vi "HandleObservation_001.vi"(8 "error in (no error)":errorcluster, 11 "S4ACS_GUI in":refnum<class "S4ACS_GUI.lvclass">) -> (0 "error out":errorcluster, 3 "S4ACS_GUI out":refnum<class "S4ACS_GUI.lvclass">)   [LabVIEW 2018, in "S4ACS_GUI.lvclass"]
uses:
  S4ACS_GUI.lvclass
  S4ACS_GUI.lvclass/S4ACS_GUI.ctl
  Instrument/Instrument.lvclass/Instrument.ctl
  Device/Optics/Optics.lvclass/Optics.ctl
  Device/Optics/Opt_Selector/Opt_Selector.lvclass
  C:/Users/observer/Desktop/Sparc4GUI/SPARC4_GUI/Device/Optics/Optics.lvclass
  Instrument/Instrument.lvclass
  StateMachine/State Machine.lvclass
  SyncBox/Sync Box.lvclass
  Trigger/Trigger.lvclass
  Acquisition/Acquisition.lvclass
  Channel/Channel.lvclass
  Device/Optics/Optics.lvclass
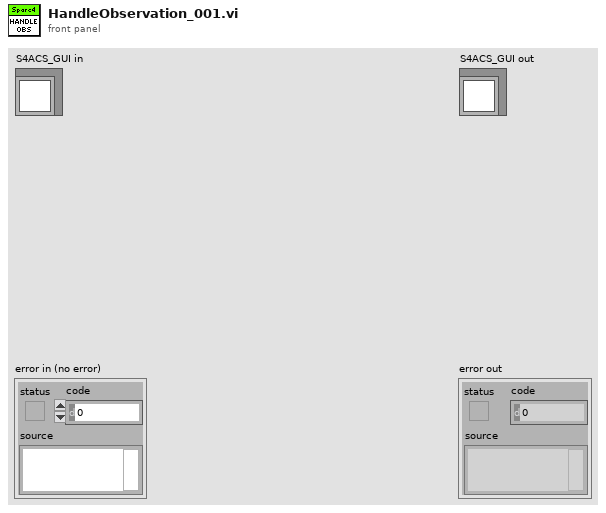
[diagram p1: front panel]
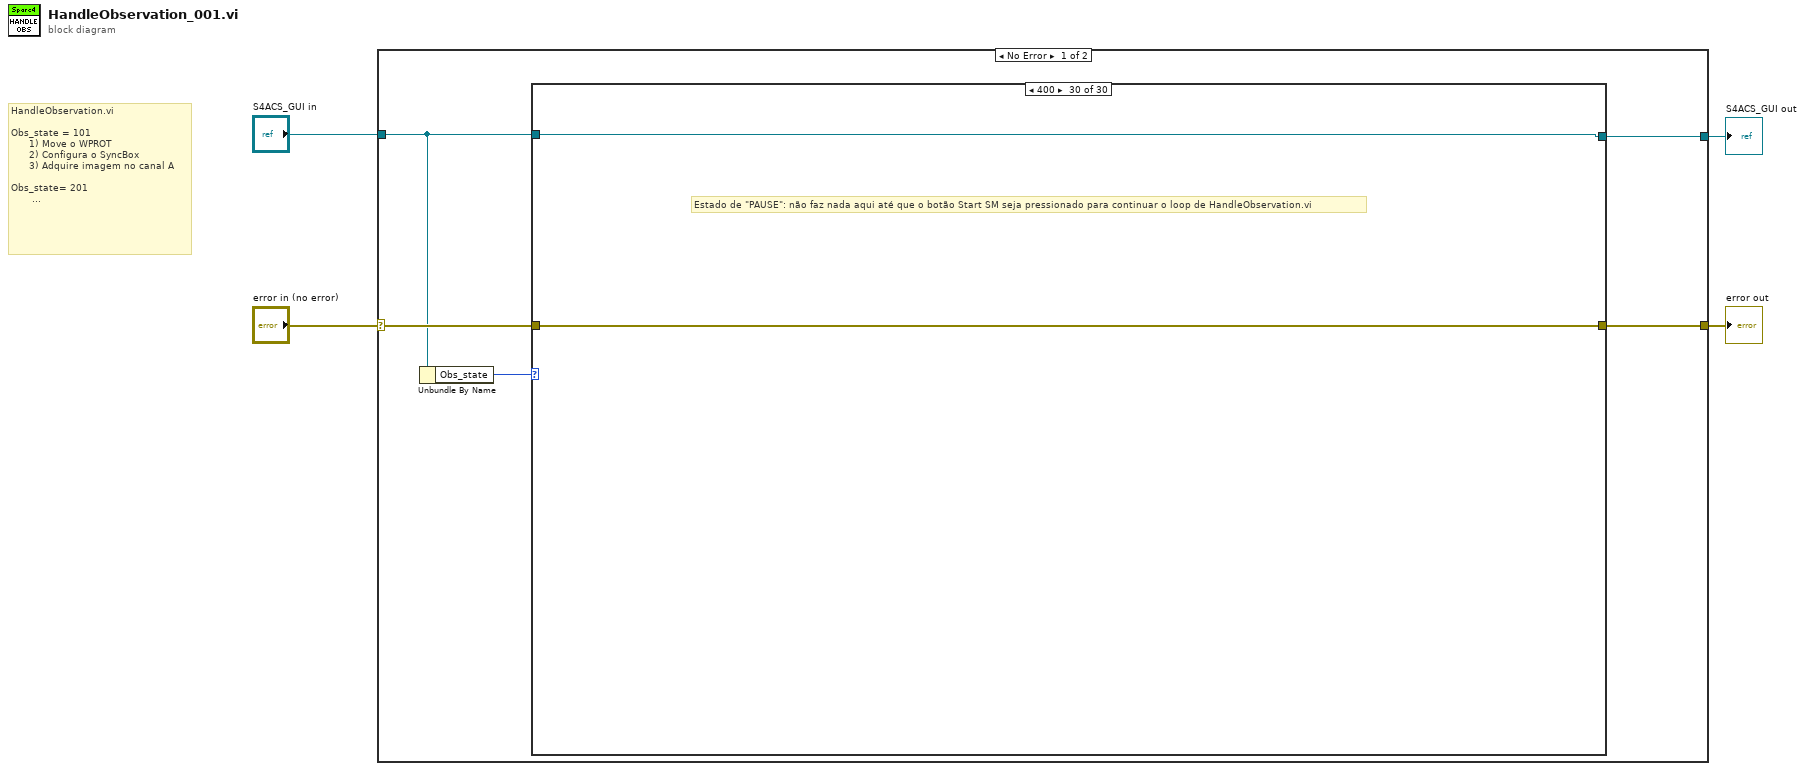
[diagram p0: block diagram]
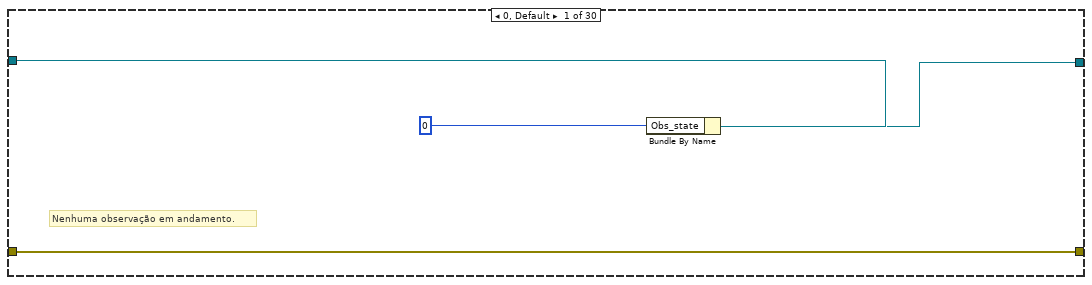
[diagram p2: hidden frame]
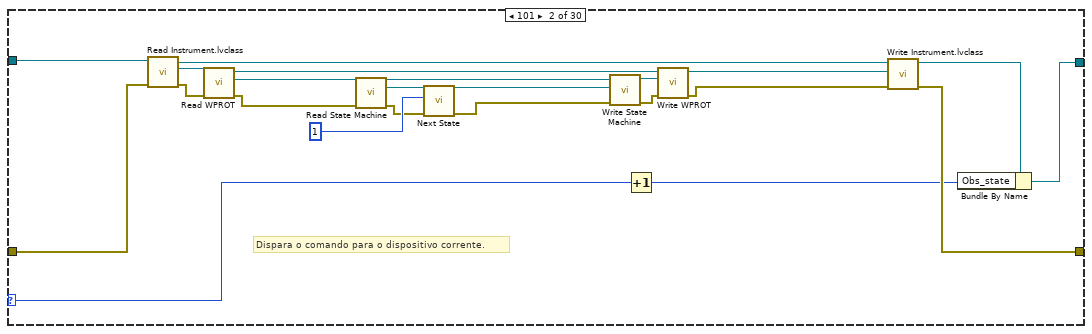
[diagram p3: hidden frame]
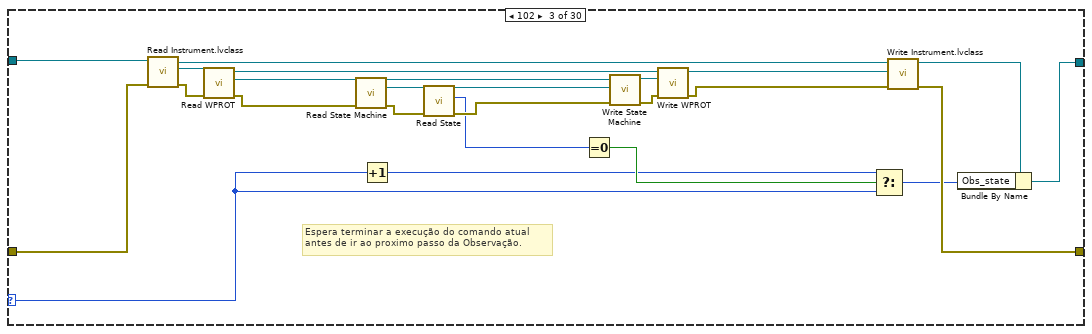
[diagram p4: hidden frame]
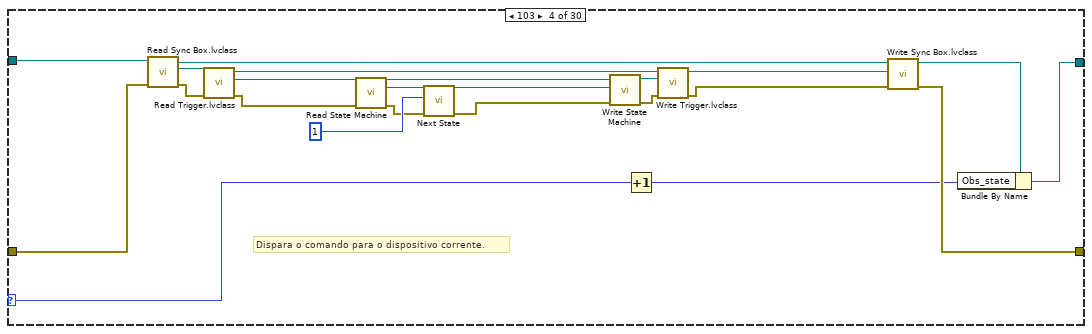
[diagram p5: hidden frame]
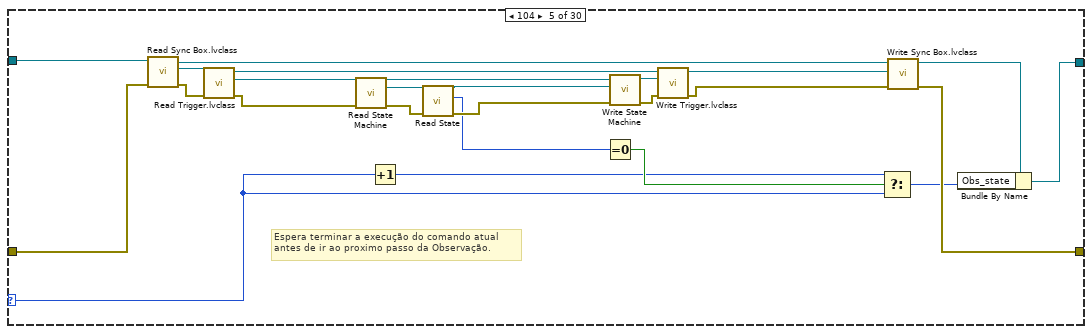
[diagram p6: hidden frame]
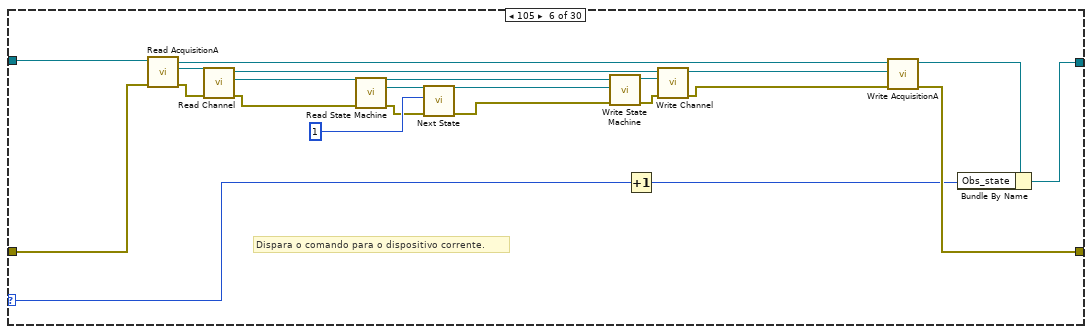
[diagram p7: hidden frame]
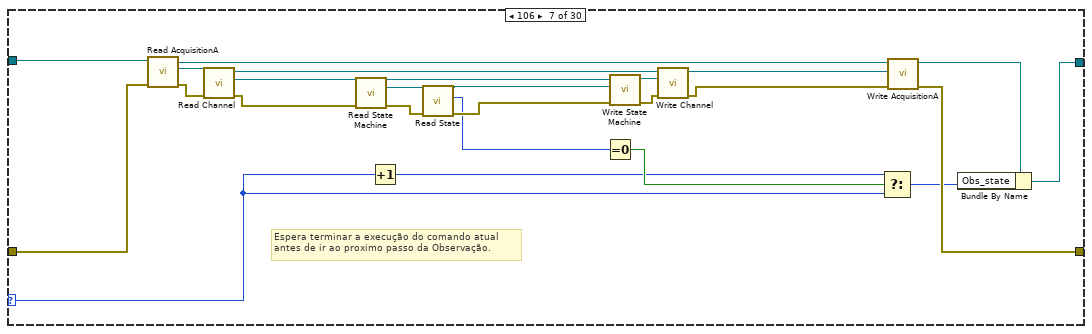
[diagram p8: hidden frame]
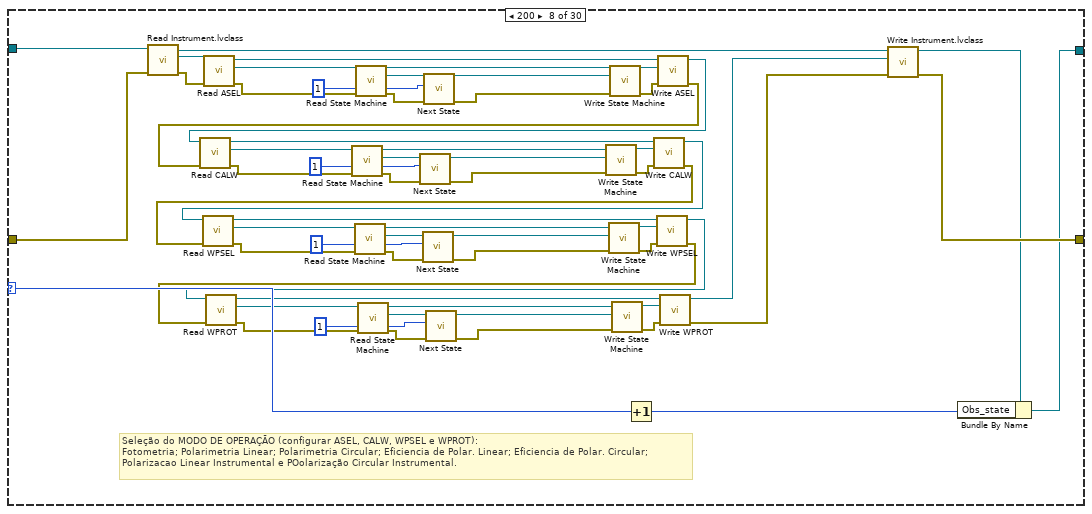
[diagram p9: hidden frame]
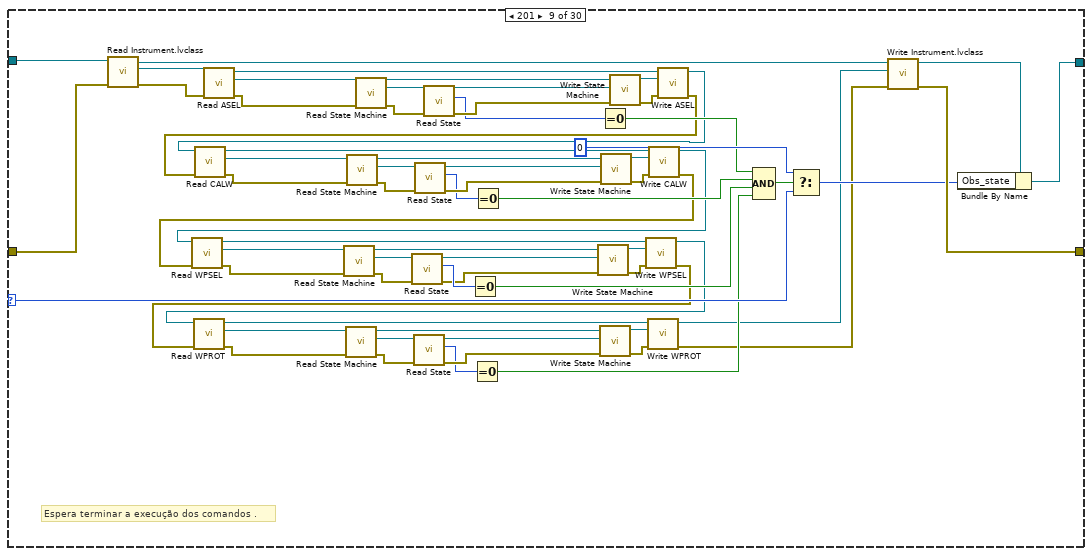
[diagram p10: hidden frame]
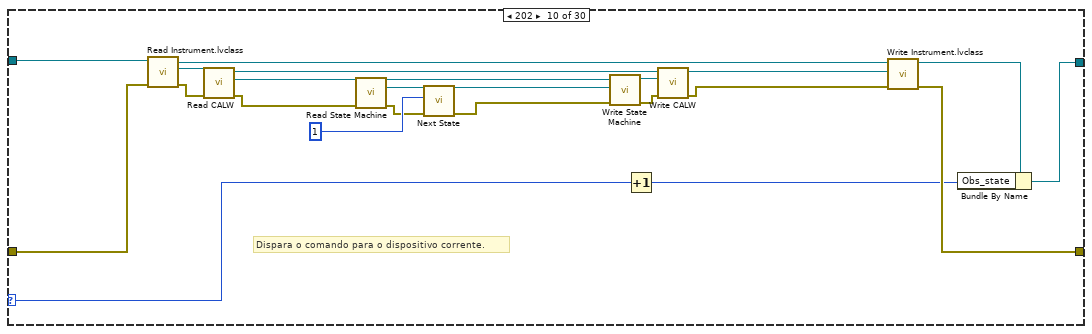
[diagram p11: hidden frame]
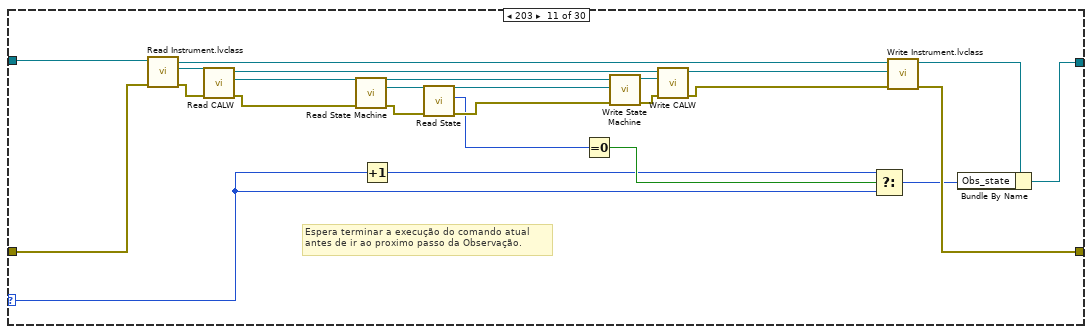
[diagram p12: hidden frame]
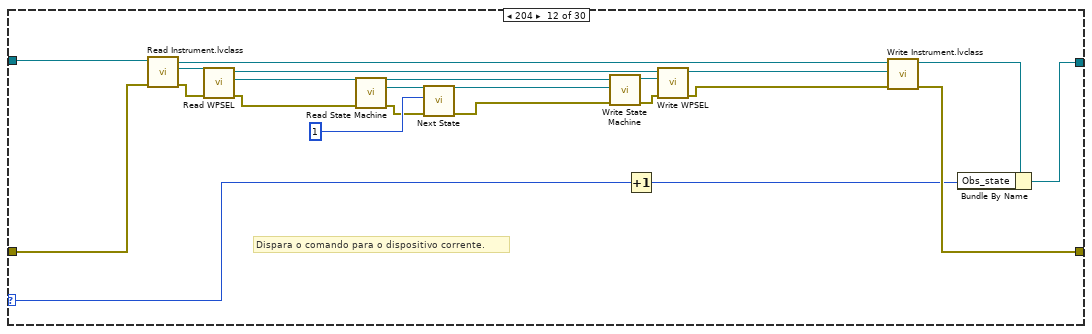
[diagram p13: hidden frame]
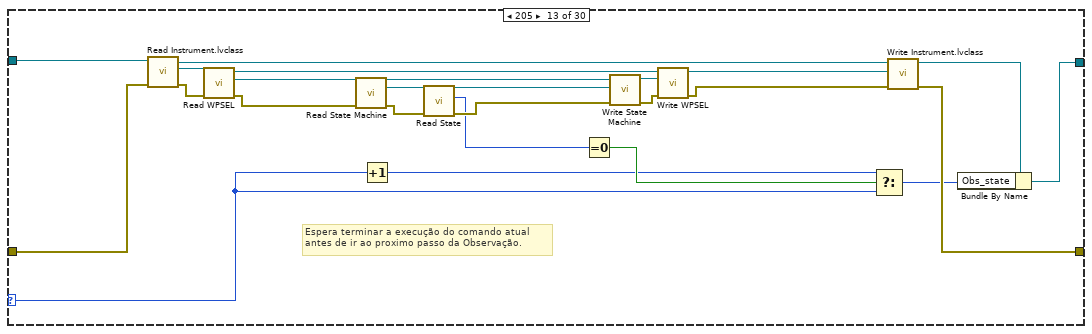
[diagram p14: hidden frame]
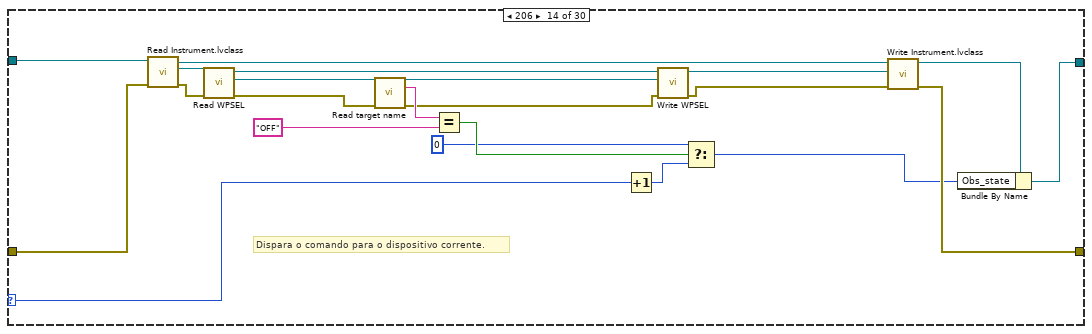
[diagram p15: hidden frame]
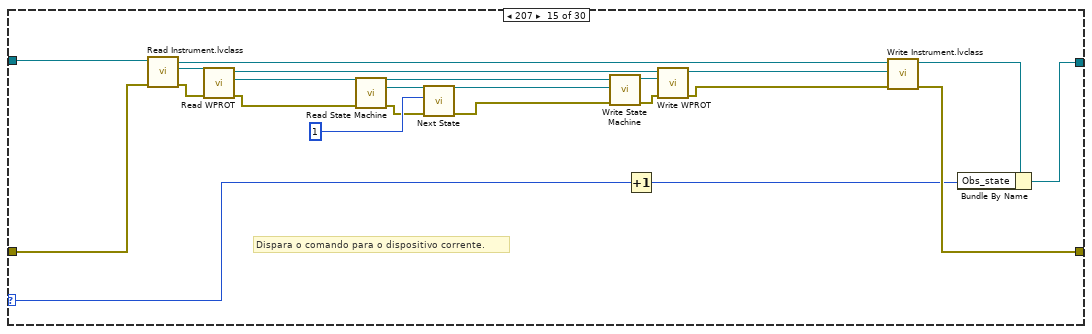
[diagram p16: hidden frame]
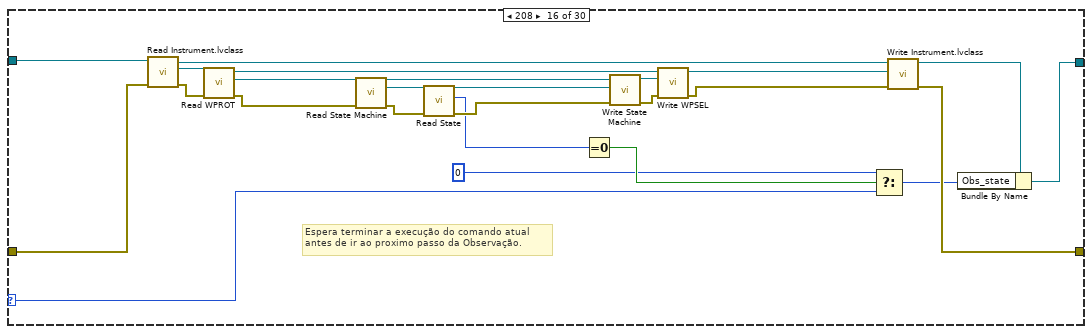
[diagram p17: hidden frame]
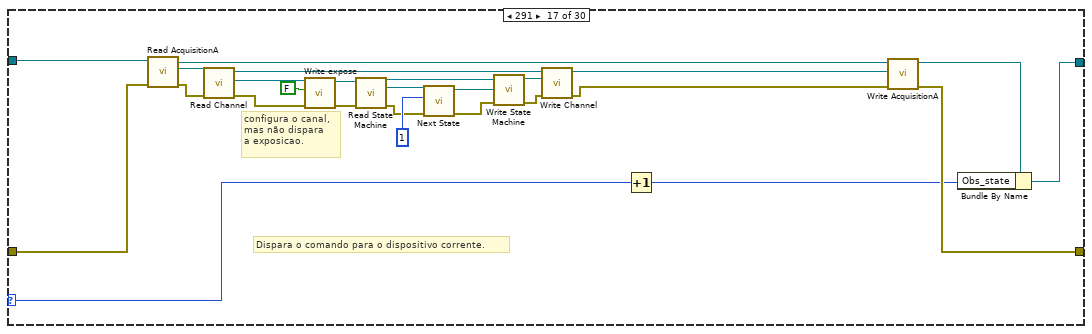
[diagram p18: hidden frame]
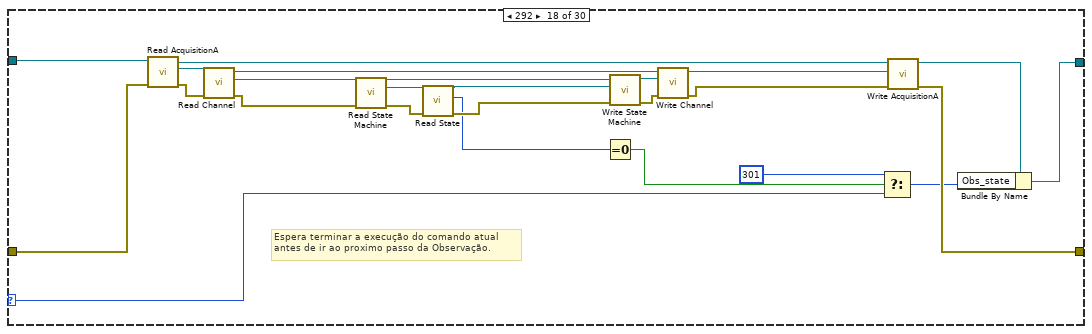
[diagram p19: hidden frame]
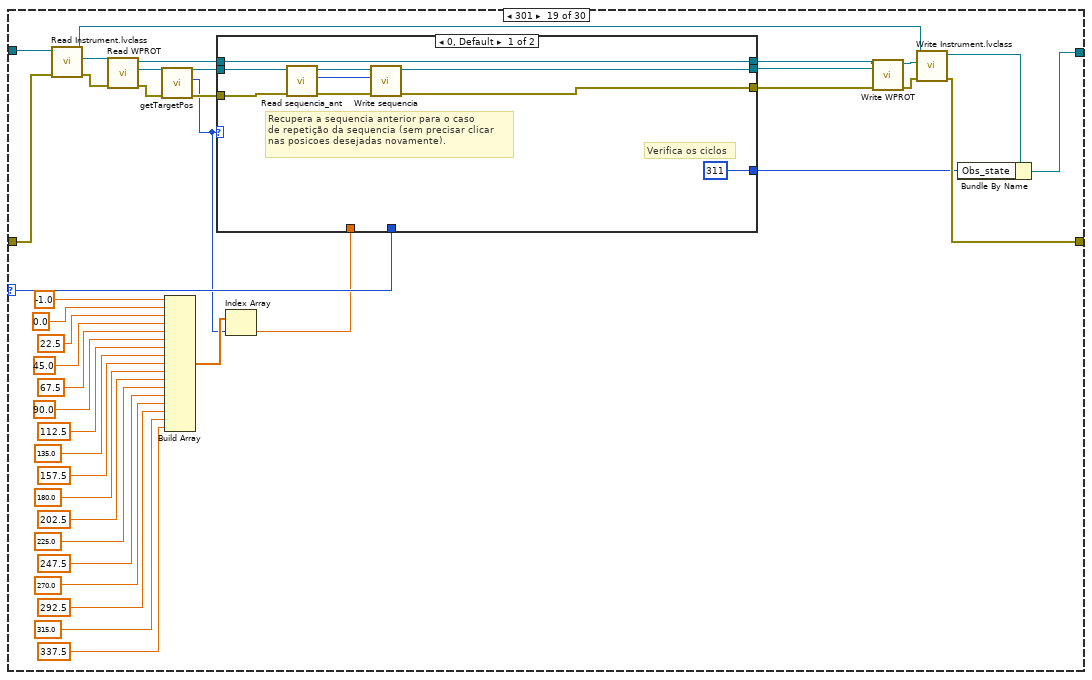
[diagram p20: hidden frame]
diagram:
  # "HandleObservation.vi\n\nObs_state = 101\n      1) Move o WPROT\n      2) Configura o SyncBox\n      3) Adquire imagem no canal A\n\nObs_state= 201\n       ..."
  n1 = case shown="No Error" "error in (no error)" {
    selector: "error in (no error)" -> [w8 w824]
    tunnel: [w7 w824] -> w3
    tunnel: [w9 w823] -> w1
    tunnel: "S4ACS_GUI in" -> [w6 w823]
    frame No Error {
      n2 = Unbundle By Name(w6) -> ("Obs_state"=w5:u32)
      n3 = case shown="400" w5 {
        selector: w5 -> [_ w16 w38 w64 w86 w112 w134 w202 w265 w290 w312 w338 w360 w395 w408 w430 w463 w482 w536 w582 w604 w636 w655 w686 w705 w734 w753 w778 _ _]
        tunnel: w6 -> [w12 w30 w55 w78 w103 w126 w151 w216 w283 w304 w329 w352 w377 w399 w422 w447 w473 w498 w540 w597 w621 w648 w672 w698 w722 w746 w770 w795 w815 w822]
        tunnel: [w10 w14 w42 w62 w94 w110 w142 w200 w270 w288 w316 w336 w364 w394 w406 w434 w461 w489 w534 w586 w612 w634 w663 w684 w713 w732 w761 w786 w811 w822] -> w9
        tunnel: w8 -> [w13 w29 w54 w77 w102 w125 w150 w215 w282 w303 w328 w351 w376 w398 w421 w446 w472 w497 w539 w596 w620 w647 w671 w697 w721 w745 w769 w794 w814 w821]
        tunnel: [w13 w28 w53 w76 w101 w124 w149 w214 w281 w302 w327 w350 w375 w397 w420 w445 w471 w496 w538 w595 w619 w646 w670 w696 w720 w744 w768 w793 w813 w821] -> w7
        frame 0, Default {
          # "Nenhuma observação em andamento."
          n4 = Bundle By Name(cluster=w12, "Obs_state"=u32 0) -> (w10:refnum<class "S4ACS_GUI.lvclass">)
        }
        frame 101 {
          # "Dispara o comando para o dispositivo corrente."
          n5 = call "Read Instrument.lvclass.vi"("error in (no error)"=w29, "S4ACS_GUI in"=w30) -> ("error out"=w35:errorcluster, "Instrument.lvclass"=w36:refnum<class "Instrument.lvclass">, "S4ACS_GUI out"=w32:refnum<class "S4ACS_GUI.lvclass">)  [unwired: 7 in]
          n6 = call "Read WPROT.vi"("error in (no error)"=w35, "Instrument in"=w36) -> ("error out"=w22:errorcluster, "Opt_Selector.lvclass"=w21:refnum<class "Opt_Selector.lvclass">, "Instrument out"=w34:refnum<class "Instrument.lvclass">)  [unwired: 7 in]
          n7 = call-dynamic "Read State Machine.vi"("error in (no error)"=w22, "Device in"=w21) -> ("error out"=w25:errorcluster, "State Machine.lvclass"=w27:refnum<class "State Machine.lvclass">, "Device out"=w19:refnum<class "Opt_Selector.lvclass">)  [unwired: 7 in]
          n8 = call "Next State.vi"("error in (no error)"=w25, "New_State"=1, "State Machine in"=w27) -> ("error out"=w24:errorcluster, "State Machine out"=w23:refnum<class "State Machine.lvclass">)  [unwired: 7 in]
          n9 = call-dynamic "Write State Machine.vi"("error in (no error)"=w24, "State Machine.lvclass"=w23, "Device in"=w19) -> ("error out"=w18:errorcluster, "Device out"=w20:refnum<class "Opt_Selector.lvclass">)  [unwired: 7 in]
          n10 = Increment(x=w16) -> (x+1=w15:u32)
          n11 = call "Write WPROT.vi"("error in (no error)"=w18, "Opt_Selector.lvclass"=w20, "Instrument in"=w34) -> ("error out"=w31:errorcluster, "Instrument out"=w33:refnum<class "Instrument.lvclass">)  [unwired: 7 in]
          n12 = call "Write Instrument.lvclass.vi"("error in (no error)"=w31, "Instrument.lvclass"=w33, "S4ACS_GUI in"=w32) -> ("error out"=w28:errorcluster, "S4ACS_GUI out"=w17:refnum<class "S4ACS_GUI.lvclass">)  [unwired: 7 in]
          n13 = Bundle By Name(cluster=w17, "Obs_state"=w15) -> (w14:refnum<class "S4ACS_GUI.lvclass">)
        }
        frame 102 {
          # "Espera terminar a execução do comando atual \nantes de ir ao proximo passo da Observação."
          n14 = call "Read Instrument.lvclass.vi"("error in (no error)"=w54, "S4ACS_GUI in"=w55) -> ("error out"=w60:errorcluster, "Instrument.lvclass"=w61:refnum<class "Instrument.lvclass">, "S4ACS_GUI out"=w57:refnum<class "S4ACS_GUI.lvclass">)  [unwired: 7 in]
          n15 = call "Read WPROT.vi"("error in (no error)"=w60, "Instrument in"=w61) -> ("error out"=w48:errorcluster, "Opt_Selector.lvclass"=w47:refnum<class "Opt_Selector.lvclass">, "Instrument out"=w59:refnum<class "Instrument.lvclass">)  [unwired: 7 in]
          n16 = call-dynamic "Read State Machine.vi"("error in (no error)"=w48, "Device in"=w47) -> ("error out"=w51:errorcluster, "State Machine.lvclass"=w52:refnum<class "State Machine.lvclass">, "Device out"=w45:refnum<class "Opt_Selector.lvclass">)  [unwired: 7 in]
          n17 = Increment(x=w38) -> (x+1=w37:u32)
          n18 = call-dynamic "Read State.vi"("error in (no error)"=w51, "State Machine in"=w52) -> ("error out"=w50:errorcluster, "State"=w40:i32, "State Machine out"=w49:refnum<class "State Machine.lvclass">)  [unwired: 7 in]
          n19 = Equal To 0?(x=w40) -> (x = 0?=w41:bool)
          n20 = call-dynamic "Write State Machine.vi"("error in (no error)"=w50, "State Machine.lvclass"=w49, "Device in"=w45) -> ("error out"=w44:errorcluster, "Device out"=w46:refnum<class "Opt_Selector.lvclass">)  [unwired: 7 in]
          n21 = call "Write WPROT.vi"("error in (no error)"=w44, "Opt_Selector.lvclass"=w46, "Instrument in"=w59) -> ("error out"=w56:errorcluster, "Instrument out"=w58:refnum<class "Instrument.lvclass">)  [unwired: 7 in]
          n22 = Select(t=w37, s=w41, f=w38) -> (s? t:f=w39:u32)
          n23 = call "Write Instrument.lvclass.vi"("error in (no error)"=w56, "Instrument.lvclass"=w58, "S4ACS_GUI in"=w57) -> ("error out"=w53:errorcluster, "S4ACS_GUI out"=w43:refnum<class "S4ACS_GUI.lvclass">)  [unwired: 7 in]
          n24 = Bundle By Name(cluster=w43, "Obs_state"=w39) -> (w42:refnum<class "S4ACS_GUI.lvclass">)
        }
        frame 103 {
          # "Dispara o comando para o dispositivo corrente."
          n25 = call-dynamic "Read Sync Box.lvclass.vi"("error in (no error)"=w77, "SPARC4_AC in"=w78) -> ("error out"=w83:errorcluster, "Sync Box.lvclass"=w84:refnum<class "Sync Box.lvclass">, "SPARC4_AC out"=w80:refnum<class "S4ACS_GUI.lvclass">)  [unwired: 7 in]
          n26 = call-dynamic "Read Trigger.lvclass.vi"("error in (no error)"=w83, "Sync Box in"=w84) -> ("error out"=w70:errorcluster, "Trigger.lvclass"=w69:refnum<class "Trigger.lvclass">, "Sync Box out"=w82:refnum<class "Sync Box.lvclass">)  [unwired: 7 in]
          n27 = call-dynamic "Read State Machine.vi"("error in (no error)"=w70, "Device in"=w69) -> ("error out"=w73:errorcluster, "State Machine.lvclass"=w75:refnum<class "State Machine.lvclass">, "Device out"=w67:refnum<class "Trigger.lvclass">)  [unwired: 7 in]
          n28 = call "Next State.vi"("error in (no error)"=w73, "New_State"=1, "State Machine in"=w75) -> ("error out"=w72:errorcluster, "State Machine out"=w71:refnum<class "State Machine.lvclass">)  [unwired: 7 in]
          n29 = call-dynamic "Write State Machine.vi"("error in (no error)"=w72, "State Machine.lvclass"=w71, "Device in"=w67) -> ("error out"=w66:errorcluster, "Device out"=w68:refnum<class "Trigger.lvclass">)  [unwired: 7 in]
          n30 = Increment(x=w64) -> (x+1=w63:u32)
          n31 = call-dynamic "Write Trigger.lvclass.vi"("error in (no error)"=w66, "Trigger.lvclass"=w68, "Sync Box in"=w82) -> ("error out"=w79:errorcluster, "Sync Box out"=w81:refnum<class "Sync Box.lvclass">)  [unwired: 7 in]
          n32 = call-dynamic "Write Sync Box.lvclass.vi"("error in (no error)"=w79, "Sync Box.lvclass"=w81, "SPARC4_AC in"=w80) -> ("error out"=w76:errorcluster, "SPARC4_AC out"=w65:refnum<class "S4ACS_GUI.lvclass">)  [unwired: 7 in]
          n33 = Bundle By Name(cluster=w65, "Obs_state"=w63) -> (w62:refnum<class "S4ACS_GUI.lvclass">)
        }
        frame 104 {
          # "Espera terminar a execução do comando atual \nantes de ir ao proximo passo da Observação."
          n34 = call-dynamic "Read Sync Box.lvclass.vi"("error in (no error)"=w102, "SPARC4_AC in"=w103) -> ("error out"=w108:errorcluster, "Sync Box.lvclass"=w109:refnum<class "Sync Box.lvclass">, "SPARC4_AC out"=w105:refnum<class "S4ACS_GUI.lvclass">)  [unwired: 7 in]
          n35 = call-dynamic "Read Trigger.lvclass.vi"("error in (no error)"=w108, "Sync Box in"=w109) -> ("error out"=w100:errorcluster, "Trigger.lvclass"=w99:refnum<class "Trigger.lvclass">, "Sync Box out"=w107:refnum<class "Sync Box.lvclass">)  [unwired: 7 in]
          n36 = call-dynamic "Read State Machine.vi"("error in (no error)"=w100, "Device in"=w99) -> ("error out"=w91:errorcluster, "State Machine.lvclass"=w93:refnum<class "State Machine.lvclass">, "Device out"=w97:refnum<class "Trigger.lvclass">)  [unwired: 7 in]
          n37 = Increment(x=w86) -> (x+1=w88:u32)
          n38 = call-dynamic "Read State.vi"("error in (no error)"=w91, "State Machine in"=w93) -> ("error out"=w90:errorcluster, "State"=w85:i32, "State Machine out"=w92:refnum<class "State Machine.lvclass">)  [unwired: 7 in]
          n39 = Equal To 0?(x=w85) -> (x = 0?=w89:bool)
          n40 = call-dynamic "Write State Machine.vi"("error in (no error)"=w90, "State Machine.lvclass"=w92, "Device in"=w97) -> ("error out"=w96:errorcluster, "Device out"=w98:refnum<class "Trigger.lvclass">)  [unwired: 7 in]
          n41 = call-dynamic "Write Trigger.lvclass.vi"("error in (no error)"=w96, "Trigger.lvclass"=w98, "Sync Box in"=w107) -> ("error out"=w104:errorcluster, "Sync Box out"=w106:refnum<class "Sync Box.lvclass">)  [unwired: 7 in]
          n42 = Select(t=w88, s=w89, f=w86) -> (s? t:f=w87:u32)
          n43 = call-dynamic "Write Sync Box.lvclass.vi"("error in (no error)"=w104, "Sync Box.lvclass"=w106, "SPARC4_AC in"=w105) -> ("error out"=w101:errorcluster, "SPARC4_AC out"=w95:refnum<class "S4ACS_GUI.lvclass">)  [unwired: 7 in]
          n44 = Bundle By Name(cluster=w95, "Obs_state"=w87) -> (w94:refnum<class "S4ACS_GUI.lvclass">)
        }
        frame 105 {
          # "Dispara o comando para o dispositivo corrente."
          n45 = call-dynamic "Read AcquisitionA.vi"("error in (no error)"=w125, "S4ACS_GUI in"=w126) -> ("error out"=w131:errorcluster, "Acquisition.lvclass"=w132:refnum<class "Acquisition.lvclass">, "S4ACS_GUI out"=w128:refnum<class "S4ACS_GUI.lvclass">)  [unwired: 7 in]
          n46 = call-dynamic "Read Channel.vi"("error in (no error)"=w131, "Acquisition in"=w132) -> ("error out"=w118:errorcluster, "Channel.lvclass"=w117:refnum<class "Channel.lvclass">, "Acquisition out"=w130:refnum<class "Acquisition.lvclass">)  [unwired: 7 in]
          n47 = call-dynamic "Read State Machine.vi"("error in (no error)"=w118, "Device in"=w117) -> ("error out"=w121:errorcluster, "State Machine.lvclass"=w123:refnum<class "State Machine.lvclass">, "Device out"=w115:refnum<class "Channel.lvclass">)  [unwired: 7 in]
          n48 = call "Next State.vi"("error in (no error)"=w121, "New_State"=1, "State Machine in"=w123) -> ("error out"=w120:errorcluster, "State Machine out"=w119:refnum<class "State Machine.lvclass">)  [unwired: 7 in]
          n49 = call-dynamic "Write State Machine.vi"("error in (no error)"=w120, "State Machine.lvclass"=w119, "Device in"=w115) -> ("error out"=w114:errorcluster, "Device out"=w116:refnum<class "Channel.lvclass">)  [unwired: 7 in]
          n50 = Increment(x=w112) -> (x+1=w111:u32)
          n51 = call-dynamic "Write Channel.vi"("error in (no error)"=w114, "Channel.lvclass"=w116, "Acquisition in"=w130) -> ("error out"=w127:errorcluster, "Acquisition out"=w129:refnum<class "Acquisition.lvclass">)  [unwired: 7 in]
          n52 = call-dynamic "Write AcquisitionA.vi"("error in (no error)"=w127, "Acquisition.lvclass"=w129, "S4ACS_GUI in"=w128) -> ("error out"=w124:errorcluster, "S4ACS_GUI out"=w113:refnum<class "S4ACS_GUI.lvclass">)  [unwired: 7 in]
          n53 = Bundle By Name(cluster=w113, "Obs_state"=w111) -> (w110:refnum<class "S4ACS_GUI.lvclass">)
        }
        frame 106 {
          # "Espera terminar a execução do comando atual \nantes de ir ao proximo passo da Observação."
          n54 = call-dynamic "Read AcquisitionA.vi"("error in (no error)"=w150, "S4ACS_GUI in"=w151) -> ("error out"=w156:errorcluster, "Acquisition.lvclass"=w157:refnum<class "Acquisition.lvclass">, "S4ACS_GUI out"=w153:refnum<class "S4ACS_GUI.lvclass">)  [unwired: 7 in]
          n55 = call-dynamic "Read Channel.vi"("error in (no error)"=w156, "Acquisition in"=w157) -> ("error out"=w148:errorcluster, "Channel.lvclass"=w147:refnum<class "Channel.lvclass">, "Acquisition out"=w155:refnum<class "Acquisition.lvclass">)  [unwired: 7 in]
          n56 = call-dynamic "Read State Machine.vi"("error in (no error)"=w148, "Device in"=w147) -> ("error out"=w139:errorcluster, "State Machine.lvclass"=w141:refnum<class "State Machine.lvclass">, "Device out"=w145:refnum<class "Channel.lvclass">)  [unwired: 7 in]
          n57 = Increment(x=w134) -> (x+1=w136:u32)
          n58 = call-dynamic "Read State.vi"("error in (no error)"=w139, "State Machine in"=w141) -> ("error out"=w138:errorcluster, "State"=w133:i32, "State Machine out"=w140:refnum<class "State Machine.lvclass">)  [unwired: 7 in]
          n59 = Equal To 0?(x=w133) -> (x = 0?=w137:bool)
          n60 = call-dynamic "Write State Machine.vi"("error in (no error)"=w138, "State Machine.lvclass"=w140, "Device in"=w145) -> ("error out"=w144:errorcluster, "Device out"=w146:refnum<class "Channel.lvclass">)  [unwired: 7 in]
          n61 = call-dynamic "Write Channel.vi"("error in (no error)"=w144, "Channel.lvclass"=w146, "Acquisition in"=w155) -> ("error out"=w152:errorcluster, "Acquisition out"=w154:refnum<class "Acquisition.lvclass">)  [unwired: 7 in]
          n62 = Select(t=w136, s=w137, f=w134) -> (s? t:f=w135:u32)
          n63 = call-dynamic "Write AcquisitionA.vi"("error in (no error)"=w152, "Acquisition.lvclass"=w154, "S4ACS_GUI in"=w153) -> ("error out"=w149:errorcluster, "S4ACS_GUI out"=w143:refnum<class "S4ACS_GUI.lvclass">)  [unwired: 7 in]
          n64 = Bundle By Name(cluster=w143, "Obs_state"=w135) -> (w142:refnum<class "S4ACS_GUI.lvclass">)
        }
        frame 200 {
          # "Seleção do MODO DE OPERAÇÃO (configurar ASEL, CALW, WPSEL e WPROT): \nFotometria; Polarimetria Linear; Polarimetria Circular; Eficiencia de Polar. Linear; Eficiencia de Polar. Circular;\nPolarizacao Linear Instrumental e POolarização Circular Instrumental."
          n65 = call "Read Instrument.lvclass.vi"("error in (no error)"=w215, "S4ACS_GUI in"=w216) -> ("error out"=w219:errorcluster, "Instrument.lvclass"=w179:refnum<class "Instrument.lvclass">, "S4ACS_GUI out"=w217:refnum<class "S4ACS_GUI.lvclass">)  [unwired: 7 in]
          n66 = call "Read ASEL.vi"("error in (no error)"=w219, "Instrument in"=w179) -> ("error out"=w208:errorcluster, "Opt_Selector.lvclass"=w207:refnum<class "Opt_Selector.lvclass">, "Instrument out"=w218:refnum<class "Instrument.lvclass">)  [unwired: 7 in]
          n67 = call-dynamic "Read State Machine.vi"("error in (no error)"=w208, "Device in"=w207) -> ("error out"=w211:errorcluster, "State Machine.lvclass"=w213:refnum<class "State Machine.lvclass">, "Device out"=w205:refnum<class "Opt_Selector.lvclass">)  [unwired: 7 in]
          n68 = call "Next State.vi"("error in (no error)"=w211, "New_State"=1, "State Machine in"=w213) -> ("error out"=w210:errorcluster, "State Machine out"=w209:refnum<class "State Machine.lvclass">)  [unwired: 7 in]
          n69 = call-dynamic "Write State Machine.vi"("error in (no error)"=w210, "State Machine.lvclass"=w209, "Device in"=w205) -> ("error out"=w204:errorcluster, "Device out"=w206:refnum<class "Opt_Selector.lvclass">)  [unwired: 7 in]
          n70 = Increment(x=w202) -> (x+1=w201:u32)
          n71 = call "Write ASEL.vi"("error in (no error)"=w204, "Opt_Selector.lvclass"=w206, "Instrument in"=w218) -> ("error out"=w160:errorcluster, "Instrument out"=w178:refnum<class "Instrument.lvclass">)  [unwired: 7 in]
          n72 = call "Read CALW.vi"("error in (no error)"=w160, "Instrument in"=w178) -> ("error out"=w195:errorcluster, "Opt_Selector.lvclass"=w196:refnum<class "Opt_Selector.lvclass">, "Instrument out"=w177:refnum<class "Instrument.lvclass">)  [unwired: 7 in]
          n73 = call-dynamic "Read State Machine.vi"("error in (no error)"=w195, "Device in"=w196) -> ("error out"=w192:errorcluster, "State Machine.lvclass"=w190:refnum<class "State Machine.lvclass">, "Device out"=w198:refnum<class "Opt_Selector.lvclass">)  [unwired: 7 in]
          n74 = call "Next State.vi"("error in (no error)"=w192, "New_State"=1, "State Machine in"=w190) -> ("error out"=w193:errorcluster, "State Machine out"=w194:refnum<class "State Machine.lvclass">)  [unwired: 7 in]
          n75 = call-dynamic "Write State Machine.vi"("error in (no error)"=w193, "State Machine.lvclass"=w194, "Device in"=w198) -> ("error out"=w199:errorcluster, "Device out"=w197:refnum<class "Opt_Selector.lvclass">)  [unwired: 7 in]
          n76 = call "Write CALW.vi"("error in (no error)"=w199, "Opt_Selector.lvclass"=w197, "Instrument in"=w177) -> ("error out"=w159:errorcluster, "Instrument out"=w176:refnum<class "Instrument.lvclass">)  [unwired: 7 in]
          n77 = call "Read WPSEL.vi"("error in (no error)"=w159, "Instrument in"=w176) -> ("error out"=w184:errorcluster, "Opt_Selector.lvclass"=w183:refnum<class "Opt_Selector.lvclass">, "Instrument out"=w175:refnum<class "Instrument.lvclass">)  [unwired: 7 in]
          n78 = call-dynamic "Read State Machine.vi"("error in (no error)"=w184, "Device in"=w183) -> ("error out"=w187:errorcluster, "State Machine.lvclass"=w189:refnum<class "State Machine.lvclass">, "Device out"=w181:refnum<class "Opt_Selector.lvclass">)  [unwired: 7 in]
          n79 = call "Next State.vi"("error in (no error)"=w187, "New_State"=1, "State Machine in"=w189) -> ("error out"=w186:errorcluster, "State Machine out"=w185:refnum<class "State Machine.lvclass">)  [unwired: 7 in]
          n80 = call-dynamic "Write State Machine.vi"("error in (no error)"=w186, "State Machine.lvclass"=w185, "Device in"=w181) -> ("error out"=w180:errorcluster, "Device out"=w182:refnum<class "Opt_Selector.lvclass">)  [unwired: 7 in]
          n81 = call "Write WPSEL.vi"("error in (no error)"=w180, "Opt_Selector.lvclass"=w182, "Instrument in"=w175) -> ("error out"=w158:errorcluster, "Instrument out"=w164:refnum<class "Instrument.lvclass">)  [unwired: 7 in]
          n82 = call "Read WPROT.vi"("error in (no error)"=w158, "Instrument in"=w164) -> ("error out"=w170:errorcluster, "Opt_Selector.lvclass"=w171:refnum<class "Opt_Selector.lvclass">, "Instrument out"=w163:refnum<class "Instrument.lvclass">)  [unwired: 7 in]
          n83 = call-dynamic "Read State Machine.vi"("error in (no error)"=w170, "Device in"=w171) -> ("error out"=w167:errorcluster, "State Machine.lvclass"=w165:refnum<class "State Machine.lvclass">, "Device out"=w173:refnum<class "Opt_Selector.lvclass">)  [unwired: 7 in]
          n84 = call "Next State.vi"("error in (no error)"=w167, "New_State"=1, "State Machine in"=w165) -> ("error out"=w168:errorcluster, "State Machine out"=w169:refnum<class "State Machine.lvclass">)  [unwired: 7 in]
          n85 = call-dynamic "Write State Machine.vi"("error in (no error)"=w168, "State Machine.lvclass"=w169, "Device in"=w173) -> ("error out"=w174:errorcluster, "Device out"=w172:refnum<class "Opt_Selector.lvclass">)  [unwired: 7 in]
          n86 = call "Write WPROT.vi"("error in (no error)"=w174, "Opt_Selector.lvclass"=w172, "Instrument in"=w163) -> ("error out"=w161:errorcluster, "Instrument out"=w162:refnum<class "Instrument.lvclass">)  [unwired: 7 in]
          n87 = call "Write Instrument.lvclass.vi"("error in (no error)"=w161, "Instrument.lvclass"=w162, "S4ACS_GUI in"=w217) -> ("error out"=w214:errorcluster, "S4ACS_GUI out"=w203:refnum<class "S4ACS_GUI.lvclass">)  [unwired: 7 in]
          n88 = Bundle By Name(cluster=w203, "Obs_state"=w201) -> (w200:refnum<class "S4ACS_GUI.lvclass">)
        }
        frame 201 {
          # "Espera terminar a execução dos comandos ."
          n89 = call "Read Instrument.lvclass.vi"("error in (no error)"=w282, "S4ACS_GUI in"=w283) -> ("error out"=w286:errorcluster, "Instrument.lvclass"=w287:refnum<class "Instrument.lvclass">, "S4ACS_GUI out"=w284:refnum<class "S4ACS_GUI.lvclass">)  [unwired: 7 in]
          n90 = call "Read ASEL.vi"("error in (no error)"=w286, "Instrument in"=w287) -> ("error out"=w276:errorcluster, "Opt_Selector.lvclass"=w275:refnum<class "Opt_Selector.lvclass">, "Instrument out"=w285:refnum<class "Instrument.lvclass">)  [unwired: 7 in]
          n91 = call-dynamic "Read State Machine.vi"("error in (no error)"=w276, "Device in"=w275) -> ("error out"=w279:errorcluster, "State Machine.lvclass"=w280:refnum<class "State Machine.lvclass">, "Device out"=w273:refnum<class "Opt_Selector.lvclass">)  [unwired: 7 in]
          n92 = call-dynamic "Read State.vi"("error in (no error)"=w279, "State Machine in"=w280) -> ("error out"=w278:errorcluster, "State"=w269:i32, "State Machine out"=w277:refnum<class "State Machine.lvclass">)  [unwired: 7 in]
          n93 = Equal To 0?(x=w269) -> (x = 0?=w264:bool)
          n94 = call-dynamic "Write State Machine.vi"("error in (no error)"=w278, "State Machine.lvclass"=w277, "Device in"=w273) -> ("error out"=w272:errorcluster, "Device out"=w274:refnum<class "Opt_Selector.lvclass">)  [unwired: 7 in]
          n95 = call "Write ASEL.vi"("error in (no error)"=w272, "Opt_Selector.lvclass"=w274, "Instrument in"=w285) -> ("error out"=w226:errorcluster, "Instrument out"=w227:refnum<class "Instrument.lvclass">)  [unwired: 7 in]
          n96 = call "Read CALW.vi"("error in (no error)"=w226, "Instrument in"=w227) -> ("error out"=w259:errorcluster, "Opt_Selector.lvclass"=w260:refnum<class "Opt_Selector.lvclass">, "Instrument out"=w230:refnum<class "Instrument.lvclass">)  [unwired: 7 in]
          n97 = call-dynamic "Read State Machine.vi"("error in (no error)"=w259, "Device in"=w260) -> ("error out"=w256:errorcluster, "State Machine.lvclass"=w255:refnum<class "State Machine.lvclass">, "Device out"=w262:refnum<class "Opt_Selector.lvclass">)  [unwired: 7 in]
          n98 = call-dynamic "Read State.vi"("error in (no error)"=w256, "State Machine in"=w255) -> ("error out"=w257:errorcluster, "State"=w254:i32, "State Machine out"=w258:refnum<class "State Machine.lvclass">)  [unwired: 7 in]
          n99 = Equal To 0?(x=w254) -> (x = 0?=w253:bool)
          n100 = call-dynamic "Write State Machine.vi"("error in (no error)"=w257, "State Machine.lvclass"=w258, "Device in"=w262) -> ("error out"=w263:errorcluster, "Device out"=w261:refnum<class "Opt_Selector.lvclass">)  [unwired: 7 in]
          n101 = call "Write CALW.vi"("error in (no error)"=w263, "Opt_Selector.lvclass"=w261, "Instrument in"=w230) -> ("error out"=w224:errorcluster, "Instrument out"=w225:refnum<class "Instrument.lvclass">)  [unwired: 7 in]
          n102 = call "Read WPSEL.vi"("error in (no error)"=w224, "Instrument in"=w225) -> ("error out"=w247:errorcluster, "Opt_Selector.lvclass"=w246:refnum<class "Opt_Selector.lvclass">, "Instrument out"=w229:refnum<class "Instrument.lvclass">)  [unwired: 7 in]
          n103 = call-dynamic "Read State Machine.vi"("error in (no error)"=w247, "Device in"=w246) -> ("error out"=w250:errorcluster, "State Machine.lvclass"=w251:refnum<class "State Machine.lvclass">, "Device out"=w244:refnum<class "Opt_Selector.lvclass">)  [unwired: 7 in]
          n104 = call-dynamic "Read State.vi"("error in (no error)"=w250, "State Machine in"=w251) -> ("error out"=w249:errorcluster, "State"=w252:i32, "State Machine out"=w248:refnum<class "State Machine.lvclass">)  [unwired: 7 in]
          n105 = Equal To 0?(x=w252) -> (x = 0?=w232:bool)
          n106 = call-dynamic "Write State Machine.vi"("error in (no error)"=w249, "State Machine.lvclass"=w248, "Device in"=w244) -> ("error out"=w243:errorcluster, "Device out"=w245:refnum<class "Opt_Selector.lvclass">)  [unwired: 7 in]
          n107 = call "Write WPSEL.vi"("error in (no error)"=w243, "Opt_Selector.lvclass"=w245, "Instrument in"=w229) -> ("error out"=w222:errorcluster, "Instrument out"=w223:refnum<class "Instrument.lvclass">)  [unwired: 7 in]
          n108 = call "Read WPROT.vi"("error in (no error)"=w222, "Instrument in"=w223) -> ("error out"=w238:errorcluster, "Opt_Selector.lvclass"=w239:refnum<class "Opt_Selector.lvclass">, "Instrument out"=w228:refnum<class "Instrument.lvclass">)  [unwired: 7 in]
          n109 = call-dynamic "Read State Machine.vi"("error in (no error)"=w238, "Device in"=w239) -> ("error out"=w235:errorcluster, "State Machine.lvclass"=w234:refnum<class "State Machine.lvclass">, "Device out"=w241:refnum<class "Opt_Selector.lvclass">)  [unwired: 7 in]
          n110 = call-dynamic "Read State.vi"("error in (no error)"=w235, "State Machine in"=w234) -> ("error out"=w236:errorcluster, "State"=w233:i32, "State Machine out"=w237:refnum<class "State Machine.lvclass">)  [unwired: 7 in]
          n111 = Equal To 0?(x=w233) -> (x = 0?=w231:bool)
          n112 = call-dynamic "Write State Machine.vi"("error in (no error)"=w236, "State Machine.lvclass"=w237, "Device in"=w241) -> ("error out"=w242:errorcluster, "Device out"=w240:refnum<class "Opt_Selector.lvclass">)  [unwired: 7 in]
          n113 = call "Write WPROT.vi"("error in (no error)"=w242, "Opt_Selector.lvclass"=w240, "Instrument in"=w228) -> ("error out"=w220:errorcluster, "Instrument out"=w221:refnum<class "Instrument.lvclass">)  [unwired: 7 in]
          n114 = Compound Arithmetic op=AND(w264, w253, w232, w231) -> (w266:bool)
          n115 = Select(t=u32 0, s=w266, f=w265) -> (s? t:f=w268:u32)
          n116 = call "Write Instrument.lvclass.vi"("error in (no error)"=w220, "Instrument.lvclass"=w221, "S4ACS_GUI in"=w284) -> ("error out"=w281:errorcluster, "S4ACS_GUI out"=w271:refnum<class "S4ACS_GUI.lvclass">)  [unwired: 7 in]
          n117 = Bundle By Name(cluster=w271, "Obs_state"=w268) -> (w270:refnum<class "S4ACS_GUI.lvclass">)
        }
        frame 202 {
          # "Dispara o comando para o dispositivo corrente."
          n118 = call "Read Instrument.lvclass.vi"("error in (no error)"=w303, "S4ACS_GUI in"=w304) -> ("error out"=w309:errorcluster, "Instrument.lvclass"=w310:refnum<class "Instrument.lvclass">, "S4ACS_GUI out"=w306:refnum<class "S4ACS_GUI.lvclass">)  [unwired: 7 in]
          n119 = call "Read CALW.vi"("error in (no error)"=w309, "Instrument in"=w310) -> ("error out"=w296:errorcluster, "Opt_Selector.lvclass"=w295:refnum<class "Opt_Selector.lvclass">, "Instrument out"=w308:refnum<class "Instrument.lvclass">)  [unwired: 7 in]
          n120 = call-dynamic "Read State Machine.vi"("error in (no error)"=w296, "Device in"=w295) -> ("error out"=w299:errorcluster, "State Machine.lvclass"=w301:refnum<class "State Machine.lvclass">, "Device out"=w293:refnum<class "Opt_Selector.lvclass">)  [unwired: 7 in]
          n121 = call "Next State.vi"("error in (no error)"=w299, "New_State"=1, "State Machine in"=w301) -> ("error out"=w298:errorcluster, "State Machine out"=w297:refnum<class "State Machine.lvclass">)  [unwired: 7 in]
          n122 = call-dynamic "Write State Machine.vi"("error in (no error)"=w298, "State Machine.lvclass"=w297, "Device in"=w293) -> ("error out"=w292:errorcluster, "Device out"=w294:refnum<class "Opt_Selector.lvclass">)  [unwired: 7 in]
          n123 = Increment(x=w290) -> (x+1=w289:u32)
          n124 = call "Write CALW.vi"("error in (no error)"=w292, "Opt_Selector.lvclass"=w294, "Instrument in"=w308) -> ("error out"=w305:errorcluster, "Instrument out"=w307:refnum<class "Instrument.lvclass">)  [unwired: 7 in]
          n125 = call "Write Instrument.lvclass.vi"("error in (no error)"=w305, "Instrument.lvclass"=w307, "S4ACS_GUI in"=w306) -> ("error out"=w302:errorcluster, "S4ACS_GUI out"=w291:refnum<class "S4ACS_GUI.lvclass">)  [unwired: 7 in]
          n126 = Bundle By Name(cluster=w291, "Obs_state"=w289) -> (w288:refnum<class "S4ACS_GUI.lvclass">)
        }
        frame 203 {
          # "Espera terminar a execução do comando atual \nantes de ir ao proximo passo da Observação."
          n127 = call "Read Instrument.lvclass.vi"("error in (no error)"=w328, "S4ACS_GUI in"=w329) -> ("error out"=w334:errorcluster, "Instrument.lvclass"=w335:refnum<class "Instrument.lvclass">, "S4ACS_GUI out"=w331:refnum<class "S4ACS_GUI.lvclass">)  [unwired: 7 in]
          n128 = call "Read CALW.vi"("error in (no error)"=w334, "Instrument in"=w335) -> ("error out"=w322:errorcluster, "Opt_Selector.lvclass"=w321:refnum<class "Opt_Selector.lvclass">, "Instrument out"=w333:refnum<class "Instrument.lvclass">)  [unwired: 7 in]
          n129 = call-dynamic "Read State Machine.vi"("error in (no error)"=w322, "Device in"=w321) -> ("error out"=w325:errorcluster, "State Machine.lvclass"=w326:refnum<class "State Machine.lvclass">, "Device out"=w319:refnum<class "Opt_Selector.lvclass">)  [unwired: 7 in]
          n130 = Increment(x=w312) -> (x+1=w311:u32)
          n131 = call-dynamic "Read State.vi"("error in (no error)"=w325, "State Machine in"=w326) -> ("error out"=w324:errorcluster, "State"=w314:i32, "State Machine out"=w323:refnum<class "State Machine.lvclass">)  [unwired: 7 in]
          n132 = Equal To 0?(x=w314) -> (x = 0?=w315:bool)
          n133 = call-dynamic "Write State Machine.vi"("error in (no error)"=w324, "State Machine.lvclass"=w323, "Device in"=w319) -> ("error out"=w318:errorcluster, "Device out"=w320:refnum<class "Opt_Selector.lvclass">)  [unwired: 7 in]
          n134 = call "Write CALW.vi"("error in (no error)"=w318, "Opt_Selector.lvclass"=w320, "Instrument in"=w333) -> ("error out"=w330:errorcluster, "Instrument out"=w332:refnum<class "Instrument.lvclass">)  [unwired: 7 in]
          n135 = Select(t=w311, s=w315, f=w312) -> (s? t:f=w313:u32)
          n136 = call "Write Instrument.lvclass.vi"("error in (no error)"=w330, "Instrument.lvclass"=w332, "S4ACS_GUI in"=w331) -> ("error out"=w327:errorcluster, "S4ACS_GUI out"=w317:refnum<class "S4ACS_GUI.lvclass">)  [unwired: 7 in]
          n137 = Bundle By Name(cluster=w317, "Obs_state"=w313) -> (w316:refnum<class "S4ACS_GUI.lvclass">)
        }
        frame 204 {
          # "Dispara o comando para o dispositivo corrente."
          n138 = call "Read Instrument.lvclass.vi"("error in (no error)"=w351, "S4ACS_GUI in"=w352) -> ("error out"=w357:errorcluster, "Instrument.lvclass"=w358:refnum<class "Instrument.lvclass">, "S4ACS_GUI out"=w354:refnum<class "S4ACS_GUI.lvclass">)  [unwired: 7 in]
          n139 = call "Read WPSEL.vi"("error in (no error)"=w357, "Instrument in"=w358) -> ("error out"=w344:errorcluster, "Opt_Selector.lvclass"=w343:refnum<class "Opt_Selector.lvclass">, "Instrument out"=w356:refnum<class "Instrument.lvclass">)  [unwired: 7 in]
          n140 = call-dynamic "Read State Machine.vi"("error in (no error)"=w344, "Device in"=w343) -> ("error out"=w347:errorcluster, "State Machine.lvclass"=w349:refnum<class "State Machine.lvclass">, "Device out"=w341:refnum<class "Opt_Selector.lvclass">)  [unwired: 7 in]
          n141 = call "Next State.vi"("error in (no error)"=w347, "New_State"=1, "State Machine in"=w349) -> ("error out"=w346:errorcluster, "State Machine out"=w345:refnum<class "State Machine.lvclass">)  [unwired: 7 in]
          n142 = call-dynamic "Write State Machine.vi"("error in (no error)"=w346, "State Machine.lvclass"=w345, "Device in"=w341) -> ("error out"=w340:errorcluster, "Device out"=w342:refnum<class "Opt_Selector.lvclass">)  [unwired: 7 in]
          n143 = Increment(x=w338) -> (x+1=w337:u32)
          n144 = call "Write WPSEL.vi"("error in (no error)"=w340, "Opt_Selector.lvclass"=w342, "Instrument in"=w356) -> ("error out"=w353:errorcluster, "Instrument out"=w355:refnum<class "Instrument.lvclass">)  [unwired: 7 in]
          n145 = call "Write Instrument.lvclass.vi"("error in (no error)"=w353, "Instrument.lvclass"=w355, "S4ACS_GUI in"=w354) -> ("error out"=w350:errorcluster, "S4ACS_GUI out"=w339:refnum<class "S4ACS_GUI.lvclass">)  [unwired: 7 in]
          n146 = Bundle By Name(cluster=w339, "Obs_state"=w337) -> (w336:refnum<class "S4ACS_GUI.lvclass">)
        }
        frame 205 {
          # "Espera terminar a execução do comando atual \nantes de ir ao proximo passo da Observação."
          n147 = call "Read Instrument.lvclass.vi"("error in (no error)"=w376, "S4ACS_GUI in"=w377) -> ("error out"=w382:errorcluster, "Instrument.lvclass"=w383:refnum<class "Instrument.lvclass">, "S4ACS_GUI out"=w379:refnum<class "S4ACS_GUI.lvclass">)  [unwired: 7 in]
          n148 = call "Read WPSEL.vi"("error in (no error)"=w382, "Instrument in"=w383) -> ("error out"=w370:errorcluster, "Opt_Selector.lvclass"=w369:refnum<class "Opt_Selector.lvclass">, "Instrument out"=w381:refnum<class "Instrument.lvclass">)  [unwired: 7 in]
          n149 = call-dynamic "Read State Machine.vi"("error in (no error)"=w370, "Device in"=w369) -> ("error out"=w373:errorcluster, "State Machine.lvclass"=w374:refnum<class "State Machine.lvclass">, "Device out"=w367:refnum<class "Opt_Selector.lvclass">)  [unwired: 7 in]
          n150 = Increment(x=w360) -> (x+1=w359:u32)
          n151 = call-dynamic "Read State.vi"("error in (no error)"=w373, "State Machine in"=w374) -> ("error out"=w372:errorcluster, "State"=w362:i32, "State Machine out"=w371:refnum<class "State Machine.lvclass">)  [unwired: 7 in]
          n152 = Equal To 0?(x=w362) -> (x = 0?=w363:bool)
          n153 = call-dynamic "Write State Machine.vi"("error in (no error)"=w372, "State Machine.lvclass"=w371, "Device in"=w367) -> ("error out"=w366:errorcluster, "Device out"=w368:refnum<class "Opt_Selector.lvclass">)  [unwired: 7 in]
          n154 = call "Write WPSEL.vi"("error in (no error)"=w366, "Opt_Selector.lvclass"=w368, "Instrument in"=w381) -> ("error out"=w378:errorcluster, "Instrument out"=w380:refnum<class "Instrument.lvclass">)  [unwired: 7 in]
          n155 = Select(t=w359, s=w363, f=w360) -> (s? t:f=w361:u32)
          n156 = call "Write Instrument.lvclass.vi"("error in (no error)"=w378, "Instrument.lvclass"=w380, "S4ACS_GUI in"=w379) -> ("error out"=w375:errorcluster, "S4ACS_GUI out"=w365:refnum<class "S4ACS_GUI.lvclass">)  [unwired: 7 in]
          n157 = Bundle By Name(cluster=w365, "Obs_state"=w361) -> (w364:refnum<class "S4ACS_GUI.lvclass">)
        }
        frame 206 {
          # "Dispara o comando para o dispositivo corrente."
          n158 = call "Read Instrument.lvclass.vi"("error in (no error)"=w398, "S4ACS_GUI in"=w399) -> ("error out"=w404:errorcluster, "Instrument.lvclass"=w405:refnum<class "Instrument.lvclass">, "S4ACS_GUI out"=w401:refnum<class "S4ACS_GUI.lvclass">)  [unwired: 7 in]
          n159 = call "Read WPSEL.vi"("error in (no error)"=w404, "Instrument in"=w405) -> ("error out"=w392:errorcluster, "Opt_Selector.lvclass"=w393:refnum<class "Opt_Selector.lvclass">, "Instrument out"=w403:refnum<class "Instrument.lvclass">)  [unwired: 7 in]
          n160 = call "Read target name.vi"("error in (no error)"=w392, "Optics in"=w393) -> ("error out"=w386:errorcluster, "target name"=w391:string, "Optics out"=w385:refnum<class "Opt_Selector.lvclass">)  [unwired: 7 in]
          n161 = Equal?(x=w391, y="OFF") -> (x = y?=w389:bool)
          n162 = Increment(x=w395) -> (x+1=w387:u32)
          n163 = call "Write WPSEL.vi"("error in (no error)"=w386, "Opt_Selector.lvclass"=w385, "Instrument in"=w403) -> ("error out"=w400:errorcluster, "Instrument out"=w402:refnum<class "Instrument.lvclass">)  [unwired: 7 in]
          n164 = Select(t=u32 0, s=w389, f=w387) -> (s? t:f=w384:u32)
          n165 = call "Write Instrument.lvclass.vi"("error in (no error)"=w400, "Instrument.lvclass"=w402, "S4ACS_GUI in"=w401) -> ("error out"=w397:errorcluster, "S4ACS_GUI out"=w396:refnum<class "S4ACS_GUI.lvclass">)  [unwired: 7 in]
          n166 = Bundle By Name(cluster=w396, "Obs_state"=w384) -> (w394:refnum<class "S4ACS_GUI.lvclass">)
        }
        frame 207 {
          # "Dispara o comando para o dispositivo corrente."
          n167 = call "Read Instrument.lvclass.vi"("error in (no error)"=w421, "S4ACS_GUI in"=w422) -> ("error out"=w427:errorcluster, "Instrument.lvclass"=w428:refnum<class "Instrument.lvclass">, "S4ACS_GUI out"=w424:refnum<class "S4ACS_GUI.lvclass">)  [unwired: 7 in]
          n168 = call "Read WPROT.vi"("error in (no error)"=w427, "Instrument in"=w428) -> ("error out"=w414:errorcluster, "Opt_Selector.lvclass"=w413:refnum<class "Opt_Selector.lvclass">, "Instrument out"=w426:refnum<class "Instrument.lvclass">)  [unwired: 7 in]
          n169 = call-dynamic "Read State Machine.vi"("error in (no error)"=w414, "Device in"=w413) -> ("error out"=w417:errorcluster, "State Machine.lvclass"=w419:refnum<class "State Machine.lvclass">, "Device out"=w411:refnum<class "Opt_Selector.lvclass">)  [unwired: 7 in]
          n170 = call "Next State.vi"("error in (no error)"=w417, "New_State"=1, "State Machine in"=w419) -> ("error out"=w416:errorcluster, "State Machine out"=w415:refnum<class "State Machine.lvclass">)  [unwired: 7 in]
          n171 = call-dynamic "Write State Machine.vi"("error in (no error)"=w416, "State Machine.lvclass"=w415, "Device in"=w411) -> ("error out"=w410:errorcluster, "Device out"=w412:refnum<class "Opt_Selector.lvclass">)  [unwired: 7 in]
          n172 = Increment(x=w408) -> (x+1=w407:u32)
          n173 = call "Write WPROT.vi"("error in (no error)"=w410, "Opt_Selector.lvclass"=w412, "Instrument in"=w426) -> ("error out"=w423:errorcluster, "Instrument out"=w425:refnum<class "Instrument.lvclass">)  [unwired: 7 in]
          n174 = call "Write Instrument.lvclass.vi"("error in (no error)"=w423, "Instrument.lvclass"=w425, "S4ACS_GUI in"=w424) -> ("error out"=w420:errorcluster, "S4ACS_GUI out"=w409:refnum<class "S4ACS_GUI.lvclass">)  [unwired: 7 in]
          n175 = Bundle By Name(cluster=w409, "Obs_state"=w407) -> (w406:refnum<class "S4ACS_GUI.lvclass">)
        }
        frame 208 {
          # "Espera terminar a execução do comando atual \nantes de ir ao proximo passo da Observação."
          n176 = call "Read Instrument.lvclass.vi"("error in (no error)"=w446, "S4ACS_GUI in"=w447) -> ("error out"=w452:errorcluster, "Instrument.lvclass"=w453:refnum<class "Instrument.lvclass">, "S4ACS_GUI out"=w449:refnum<class "S4ACS_GUI.lvclass">)  [unwired: 7 in]
          n177 = call "Read WPROT.vi"("error in (no error)"=w452, "Instrument in"=w453) -> ("error out"=w440:errorcluster, "Opt_Selector.lvclass"=w439:refnum<class "Opt_Selector.lvclass">, "Instrument out"=w451:refnum<class "Instrument.lvclass">)  [unwired: 7 in]
          n178 = call-dynamic "Read State Machine.vi"("error in (no error)"=w440, "Device in"=w439) -> ("error out"=w443:errorcluster, "State Machine.lvclass"=w444:refnum<class "State Machine.lvclass">, "Device out"=w437:refnum<class "Opt_Selector.lvclass">)  [unwired: 7 in]
          n179 = call-dynamic "Read State.vi"("error in (no error)"=w443, "State Machine in"=w444) -> ("error out"=w442:errorcluster, "State"=w432:i32, "State Machine out"=w441:refnum<class "State Machine.lvclass">)  [unwired: 7 in]
          n180 = Equal To 0?(x=w432) -> (x = 0?=w433:bool)
          n181 = call-dynamic "Write State Machine.vi"("error in (no error)"=w442, "State Machine.lvclass"=w441, "Device in"=w437) -> ("error out"=w436:errorcluster, "Device out"=w438:refnum<class "Opt_Selector.lvclass">)  [unwired: 7 in]
          n182 = call "Write WPSEL.vi"("error in (no error)"=w436, "Opt_Selector.lvclass"=w438, "Instrument in"=w451) -> ("error out"=w448:errorcluster, "Instrument out"=w450:refnum<class "Instrument.lvclass">)  [unwired: 7 in]
          n183 = Select(t=u32 0, s=w433, f=w430) -> (s? t:f=w431:u32)
          n184 = call "Write Instrument.lvclass.vi"("error in (no error)"=w448, "Instrument.lvclass"=w450, "S4ACS_GUI in"=w449) -> ("error out"=w445:errorcluster, "S4ACS_GUI out"=w435:refnum<class "S4ACS_GUI.lvclass">)  [unwired: 7 in]
          n185 = Bundle By Name(cluster=w435, "Obs_state"=w431) -> (w434:refnum<class "S4ACS_GUI.lvclass">)
        }
        frame 291 {
          # "configura o canal,\nmas não dispara\na exposicao."
          # "Dispara o comando para o dispositivo corrente."
          n186 = call-dynamic "Read AcquisitionA.vi"("error in (no error)"=w472, "S4ACS_GUI in"=w473) -> ("error out"=w478:errorcluster, "Acquisition.lvclass"=w479:refnum<class "Acquisition.lvclass">, "S4ACS_GUI out"=w475:refnum<class "S4ACS_GUI.lvclass">)  [unwired: 7 in]
          n187 = call-dynamic "Read Channel.vi"("error in (no error)"=w478, "Acquisition in"=w479) -> ("error out"=w458:errorcluster, "Channel.lvclass"=w460:refnum<class "Channel.lvclass">, "Acquisition out"=w477:refnum<class "Acquisition.lvclass">)  [unwired: 7 in]
          n188 = call-dynamic "Write expose.vi"("error in (no error)"=w458, "expose"=FALSE, "Channel in"=w460) -> ("error out"=w457:errorcluster, "Channel out"=w459:refnum<class "Channel.lvclass">)  [unwired: 7 in]
          n189 = call-dynamic "Read State Machine.vi"("error in (no error)"=w457, "Device in"=w459) -> ("error out"=w468:errorcluster, "State Machine.lvclass"=w470:refnum<class "State Machine.lvclass">, "Device out"=w466:refnum<class "Channel.lvclass">)  [unwired: 7 in]
          n190 = call "Next State.vi"("error in (no error)"=w468, "New_State"=1, "State Machine in"=w470) -> ("error out"=w454:errorcluster, "State Machine out"=w455:refnum<class "State Machine.lvclass">)  [unwired: 7 in]
          n191 = call-dynamic "Write State Machine.vi"("error in (no error)"=w454, "State Machine.lvclass"=w455, "Device in"=w466) -> ("error out"=w465:errorcluster, "Device out"=w467:refnum<class "Channel.lvclass">)  [unwired: 7 in]
          n192 = call-dynamic "Write Channel.vi"("error in (no error)"=w465, "Channel.lvclass"=w467, "Acquisition in"=w477) -> ("error out"=w474:errorcluster, "Acquisition out"=w476:refnum<class "Acquisition.lvclass">)  [unwired: 7 in]
          n193 = Increment(x=w463) -> (x+1=w462:u32)
          n194 = call-dynamic "Write AcquisitionA.vi"("error in (no error)"=w474, "Acquisition.lvclass"=w476, "S4ACS_GUI in"=w475) -> ("error out"=w471:errorcluster, "S4ACS_GUI out"=w464:refnum<class "S4ACS_GUI.lvclass">)  [unwired: 7 in]
          n195 = Bundle By Name(cluster=w464, "Obs_state"=w462) -> (w461:refnum<class "S4ACS_GUI.lvclass">)
        }
        frame 292 {
          # "Espera terminar a execução do comando atual \nantes de ir ao proximo passo da Observação."
          n196 = call-dynamic "Read AcquisitionA.vi"("error in (no error)"=w497, "S4ACS_GUI in"=w498) -> ("error out"=w503:errorcluster, "Acquisition.lvclass"=w504:refnum<class "Acquisition.lvclass">, "S4ACS_GUI out"=w500:refnum<class "S4ACS_GUI.lvclass">)  [unwired: 7 in]
          n197 = call-dynamic "Read Channel.vi"("error in (no error)"=w503, "Acquisition in"=w504) -> ("error out"=w495:errorcluster, "Channel.lvclass"=w494:refnum<class "Channel.lvclass">, "Acquisition out"=w502:refnum<class "Acquisition.lvclass">)  [unwired: 7 in]
          n198 = call-dynamic "Read State Machine.vi"("error in (no error)"=w495, "Device in"=w494) -> ("error out"=w486:errorcluster, "State Machine.lvclass"=w488:refnum<class "State Machine.lvclass">, "Device out"=w492:refnum<class "Channel.lvclass">)  [unwired: 7 in]
          n199 = call-dynamic "Read State.vi"("error in (no error)"=w486, "State Machine in"=w488) -> ("error out"=w485:errorcluster, "State"=w481:i32, "State Machine out"=w487:refnum<class "State Machine.lvclass">)  [unwired: 7 in]
          n200 = Equal To 0?(x=w481) -> (x = 0?=w484:bool)
          n201 = call-dynamic "Write State Machine.vi"("error in (no error)"=w485, "State Machine.lvclass"=w487, "Device in"=w492) -> ("error out"=w491:errorcluster, "Device out"=w493:refnum<class "Channel.lvclass">)  [unwired: 7 in]
          n202 = call-dynamic "Write Channel.vi"("error in (no error)"=w491, "Channel.lvclass"=w493, "Acquisition in"=w502) -> ("error out"=w499:errorcluster, "Acquisition out"=w501:refnum<class "Acquisition.lvclass">)  [unwired: 7 in]
          n203 = Select(t=u32 301, s=w484, f=w482) -> (s? t:f=w483:u32)
          n204 = call-dynamic "Write AcquisitionA.vi"("error in (no error)"=w499, "Acquisition.lvclass"=w501, "S4ACS_GUI in"=w500) -> ("error out"=w496:errorcluster, "S4ACS_GUI out"=w490:refnum<class "S4ACS_GUI.lvclass">)  [unwired: 7 in]
          n205 = Bundle By Name(cluster=w490, "Obs_state"=w483) -> (w489:refnum<class "S4ACS_GUI.lvclass">)
        }
        frame 301 {
          n206 = call "Read Instrument.lvclass.vi"("error in (no error)"=w539, "S4ACS_GUI in"=w540) -> ("error out"=w543:errorcluster, "Instrument.lvclass"=w544:refnum<class "Instrument.lvclass">, "S4ACS_GUI out"=w541:refnum<class "S4ACS_GUI.lvclass">)  [unwired: 7 in]
          n207 = call "Read WPROT.vi"("error in (no error)"=w543, "Instrument in"=w544) -> ("error out"=w532:errorcluster, "Opt_Selector.lvclass"=w533:refnum<class "Opt_Selector.lvclass">, "Instrument out"=w542:refnum<class "Instrument.lvclass">)  [unwired: 7 in]
          n208 = call-dynamic "getTargetPos.vi"("error in (no error)"=w532, "Opt_Selector in"=w533) -> ("error out"=w531:errorcluster, "Target Pos"=w511:u16, "Opt_Selector out"=w530:refnum<class "Opt_Selector.lvclass">)  [unwired: 7 in]
          n209 = Build Array(-1.0 ("element"), 0.0 ("element"), 22.5 ("element"), 45.0 ("element"), 67.5 ("element"), 90.0 ("element"), 112.5 ("element"), 135.0 ("element"), 157.5 ("element"), 180.0 ("element"), 202.5 ("element"), 225.0 ("element"), 247.5 ("element"), 270.0 ("element"), 292.5 ("element"), 315.0 ("element"), 337.5 ("element")) -> (w523:dbl[])
          n210 = Index Array(array=w523, index=w511) -> (element=w510:dbl)
          n211 = case shown="0, Default" w511 {
            selector: w511 -> [_ w567]
            tunnel: w542 -> [w552 w555]
            tunnel: [w552 w555] -> w506
            tunnel: [w549 w554] -> w505
            tunnel: w536 -> [_ w569]
            tunnel: [u32 311 w568] -> w535
            tunnel: w531 -> [w550 w563]
            tunnel: w530 -> [w551 w562]
            tunnel: w510 -> [_ w557]
            tunnel: [w547 w556] -> w507
            frame 0, Default {
              # "Verifica os ciclos"
              # "Recupera a sequencia anterior para o caso \nde repetição da sequencia (sem precisar clicar \nnas posicoes desejadas novamente)."
              n212 = call-dynamic "Read sequencia_ant.vi"("error in (no error)"=w550, "Opt_Selector in"=w551) -> ("error out"=w546:errorcluster, "sequencia_ant"=w545:u16, "Opt_Selector out"=w548:refnum<class "Opt_Selector.lvclass">)  [unwired: 7 in]
              n213 = call-dynamic "Write sequencia.vi"("error in (no error)"=w546, "sequencia"=w545, "Opt_Selector in"=w548) -> ("error out"=w549:errorcluster, "Opt_Selector out"=w547:refnum<class "Opt_Selector.lvclass">)  [unwired: 7 in]
            }
            frame 1..16 {
              n214 = Number To Decimal String(number=w567) -> (decimal integer string=w566:string)  [unwired: 1 in]
              n215 = Concatenate Strings("WP" ("string"), w566) -> (w564:string)
              n216 = call "Write target name.vi"("error in (no error)"=w563, "target name"=w564, "Optics in"=w562) -> ("error out"=w560:errorcluster, "Optics out"=w561:refnum<class "Opt_Selector.lvclass">)  [unwired: 7 in]
              n217 = call "Write target.vi"("error in (no error)"=w560, "target"=w557, "Optics in"=w561) -> ("error out"=w559:errorcluster, "Optics out"=w558:refnum<class "Opt_Selector.lvclass">)  [unwired: 7 in]
              n218 = call-dynamic "Read State Machine.vi"("error in (no error)"=w559, "Device in"=w558) -> ("error out"=w573:errorcluster, "State Machine.lvclass"=w575:refnum<class "State Machine.lvclass">, "Device out"=w570:refnum<class "Opt_Selector.lvclass">)  [unwired: 7 in]
              n219 = Increment(x=w569) -> (x+1=w568:u32)
              n220 = call "Next State.vi"("error in (no error)"=w573, "New_State"=1, "State Machine in"=w575) -> ("error out"=w572:errorcluster, "State Machine out"=w571:refnum<class "State Machine.lvclass">)  [unwired: 7 in]
              n221 = call-dynamic "Write State Machine.vi"("error in (no error)"=w572, "State Machine.lvclass"=w571, "Device in"=w570) -> ("error out"=w554:errorcluster, "Device out"=w556:refnum<class "Opt_Selector.lvclass">)  [unwired: 7 in]
            }
          }
          n222 = call "Write WPROT.vi"("error in (no error)"=w505, "Opt_Selector.lvclass"=w507, "Instrument in"=w506) -> ("error out"=w509:errorcluster, "Instrument out"=w508:refnum<class "Instrument.lvclass">)  [unwired: 7 in]
          n223 = call "Write Instrument.lvclass.vi"("error in (no error)"=w509, "Instrument.lvclass"=w508, "S4ACS_GUI in"=w541) -> ("error out"=w538:errorcluster, "S4ACS_GUI out"=w537:refnum<class "S4ACS_GUI.lvclass">)  [unwired: 7 in]
          n224 = Bundle By Name(cluster=w537, "Obs_state"=w535) -> (w534:refnum<class "S4ACS_GUI.lvclass">)
        }
        frame 302 {
          # "TESTE: 1 x 20ms = 0.02s de pausa entre \nposições do waveplate."
          # "Espera terminar o movimento para a posição \"target\" do waveplate\nantes de ir para o estado de pausa."
          n225 = call "Read Instrument.lvclass.vi"("error in (no error)"=w596, "S4ACS_GUI in"=w597) -> ("error out"=w602:errorcluster, "Instrument.lvclass"=w603:refnum<class "Instrument.lvclass">, "S4ACS_GUI out"=w599:refnum<class "S4ACS_GUI.lvclass">)  [unwired: 7 in]
          n226 = call "Read WPROT.vi"("error in (no error)"=w602, "Instrument in"=w603) -> ("error out"=w592:errorcluster, "Opt_Selector.lvclass"=w591:refnum<class "Opt_Selector.lvclass">, "Instrument out"=w601:refnum<class "Instrument.lvclass">)  [unwired: 7 in]
          n227 = call-dynamic "Read State Machine.vi"("error in (no error)"=w592, "Device in"=w591) -> ("error out"=w593:errorcluster, "State Machine.lvclass"=w594:refnum<class "State Machine.lvclass">, "Device out"=w589:refnum<class "Opt_Selector.lvclass">)  [unwired: 7 in]
          n228 = Increment(x=w582) -> (x+1=w581:u32)
          n229 = call-dynamic "Read State.vi"("error in (no error)"=w593, "State Machine in"=w594) -> ("error out"=w576:errorcluster, "State"=w584:i32, "State Machine out"=w580:refnum<class "State Machine.lvclass">)  [unwired: 7 in]
          n230 = Equal To 0?(x=w584) -> (x = 0?=w585:bool)
          n231 = call-dynamic "Write Timer.vi"("error in (no error)"=w576, "Timer"=u32 1, "State Machine in"=w580) -> ("error out"=w577:errorcluster, "State Machine out"=w579:refnum<class "State Machine.lvclass">)  [unwired: 7 in]
          n232 = call-dynamic "Write State Machine.vi"("error in (no error)"=w577, "State Machine.lvclass"=w579, "Device in"=w589) -> ("error out"=w588:errorcluster, "Device out"=w590:refnum<class "Opt_Selector.lvclass">)  [unwired: 7 in]
          n233 = call "Write WPROT.vi"("error in (no error)"=w588, "Opt_Selector.lvclass"=w590, "Instrument in"=w601) -> ("error out"=w598:errorcluster, "Instrument out"=w600:refnum<class "Instrument.lvclass">)  [unwired: 7 in]
          n234 = Select(t=w581, s=w585, f=w582) -> (s? t:f=w583:u32)
          n235 = call "Write Instrument.lvclass.vi"("error in (no error)"=w598, "Instrument.lvclass"=w600, "S4ACS_GUI in"=w599) -> ("error out"=w595:errorcluster, "S4ACS_GUI out"=w587:refnum<class "S4ACS_GUI.lvclass">)  [unwired: 7 in]
          n236 = Bundle By Name(cluster=w587, "Obs_state"=w583) -> (w586:refnum<class "S4ACS_GUI.lvclass">)
        }
        frame 303 {
          # "Espera terminar a pausa carregada no Timer"
          n237 = call "Read Instrument.lvclass.vi"("error in (no error)"=w620, "S4ACS_GUI in"=w621) -> ("error out"=w626:errorcluster, "Instrument.lvclass"=w627:refnum<class "Instrument.lvclass">, "S4ACS_GUI out"=w623:refnum<class "S4ACS_GUI.lvclass">)  [unwired: 7 in]
          n238 = call "Read WPROT.vi"("error in (no error)"=w626, "Instrument in"=w627) -> ("error out"=w618:errorcluster, "Opt_Selector.lvclass"=w617:refnum<class "Opt_Selector.lvclass">, "Instrument out"=w625:refnum<class "Instrument.lvclass">)  [unwired: 7 in]
          n239 = call-dynamic "Read State Machine.vi"("error in (no error)"=w618, "Device in"=w617) -> ("error out"=w607:errorcluster, "State Machine.lvclass"=w608:refnum<class "State Machine.lvclass">, "Device out"=w615:refnum<class "Opt_Selector.lvclass">)  [unwired: 7 in]
          n240 = Increment(x=w604) -> (x+1=w609:u32)
          n241 = call "Verify Timer.vi"("error in (no error)"=w607, "State Machine in"=w608) -> ("error out"=w605:errorcluster, "timeout"=w610:bool, "State Machine out"=w606:refnum<class "State Machine.lvclass">)  [unwired: 7 in]
          n242 = call-dynamic "Write State Machine.vi"("error in (no error)"=w605, "State Machine.lvclass"=w606, "Device in"=w615) -> ("error out"=w614:errorcluster, "Device out"=w616:refnum<class "Opt_Selector.lvclass">)  [unwired: 7 in]
          n243 = call "Write WPROT.vi"("error in (no error)"=w614, "Opt_Selector.lvclass"=w616, "Instrument in"=w625) -> ("error out"=w622:errorcluster, "Instrument out"=w624:refnum<class "Instrument.lvclass">)  [unwired: 7 in]
          n244 = call "Write Instrument.lvclass.vi"("error in (no error)"=w622, "Instrument.lvclass"=w624, "S4ACS_GUI in"=w623) -> ("error out"=w619:errorcluster, "S4ACS_GUI out"=w613:refnum<class "S4ACS_GUI.lvclass">)  [unwired: 7 in]
          n245 = Select(t=w609, s=w610, f=w604) -> (s? t:f=w611:u32)
          n246 = Bundle By Name(cluster=w613, "Obs_state"=w611) -> (w612:refnum<class "S4ACS_GUI.lvclass">)
        }
        frame 304 {
          # "configura delays do syncBox"
          # "Dispara o comando para o dispositivo corrente."
          n247 = call-dynamic "Read Sync Box.lvclass.vi"("error in (no error)"=w647, "SPARC4_AC in"=w648) -> ("error out"=w653:errorcluster, "Sync Box.lvclass"=w628:refnum<class "Sync Box.lvclass">, "SPARC4_AC out"=w650:refnum<class "S4ACS_GUI.lvclass">)  [unwired: 7 in]
          n248 = call-dynamic "Read Trigger.lvclass.vi"("error in (no error)"=w653, "Sync Box in"=w628) -> ("error out"=w642:errorcluster, "Trigger.lvclass"=w641:refnum<class "Trigger.lvclass">, "Sync Box out"=w652:refnum<class "Sync Box.lvclass">)  [unwired: 7 in]
          n249 = call-dynamic "Read State Machine.vi"("error in (no error)"=w642, "Device in"=w641) -> ("error out"=w643:errorcluster, "State Machine.lvclass"=w645:refnum<class "State Machine.lvclass">, "Device out"=w639:refnum<class "Trigger.lvclass">)  [unwired: 7 in]
          n250 = call "Next State.vi"("error in (no error)"=w643, "New_State"=10, "State Machine in"=w645) -> ("error out"=w630:errorcluster, "State Machine out"=w632:refnum<class "State Machine.lvclass">)  [unwired: 7 in]
          n251 = call-dynamic "Write Timer.vi"("error in (no error)"=w630, "Timer"=u32 5, "State Machine in"=w632) -> ("error out"=w629:errorcluster, "State Machine out"=w631:refnum<class "State Machine.lvclass">)  [unwired: 7 in]
          n252 = call-dynamic "Write State Machine.vi"("error in (no error)"=w629, "State Machine.lvclass"=w631, "Device in"=w639) -> ("error out"=w638:errorcluster, "Device out"=w640:refnum<class "Trigger.lvclass">)  [unwired: 7 in]
          n253 = Increment(x=w636) -> (x+1=w635:u32)
          n254 = call-dynamic "Write Trigger.lvclass.vi"("error in (no error)"=w638, "Trigger.lvclass"=w640, "Sync Box in"=w652) -> ("error out"=w649:errorcluster, "Sync Box out"=w651:refnum<class "Sync Box.lvclass">)  [unwired: 7 in]
          n255 = call-dynamic "Write Sync Box.lvclass.vi"("error in (no error)"=w649, "Sync Box.lvclass"=w651, "SPARC4_AC in"=w650) -> ("error out"=w646:errorcluster, "SPARC4_AC out"=w637:refnum<class "S4ACS_GUI.lvclass">)  [unwired: 7 in]
          n256 = Bundle By Name(cluster=w637, "Obs_state"=w635) -> (w634:refnum<class "S4ACS_GUI.lvclass">)
        }
        frame 305 {
          # "Espera terminar a execução do comando atual \nantes de ir ao proximo passo da Observação."
          n257 = call-dynamic "Read Sync Box.lvclass.vi"("error in (no error)"=w671, "SPARC4_AC in"=w672) -> ("error out"=w677:errorcluster, "Sync Box.lvclass"=w678:refnum<class "Sync Box.lvclass">, "SPARC4_AC out"=w674:refnum<class "S4ACS_GUI.lvclass">)  [unwired: 7 in]
          n258 = call-dynamic "Read Trigger.lvclass.vi"("error in (no error)"=w677, "Sync Box in"=w678) -> ("error out"=w669:errorcluster, "Trigger.lvclass"=w668:refnum<class "Trigger.lvclass">, "Sync Box out"=w676:refnum<class "Sync Box.lvclass">)  [unwired: 7 in]
          n259 = call-dynamic "Read State Machine.vi"("error in (no error)"=w669, "Device in"=w668) -> ("error out"=w660:errorcluster, "State Machine.lvclass"=w662:refnum<class "State Machine.lvclass">, "Device out"=w666:refnum<class "Trigger.lvclass">)  [unwired: 7 in]
          n260 = call-dynamic "Read State.vi"("error in (no error)"=w660, "State Machine in"=w662) -> ("error out"=w659:errorcluster, "State"=w656:i32, "State Machine out"=w661:refnum<class "State Machine.lvclass">)  [unwired: 7 in]
          n261 = Equal To 0?(x=w656) -> (x = 0?=w658:bool)
          n262 = call-dynamic "Write State Machine.vi"("error in (no error)"=w659, "State Machine.lvclass"=w661, "Device in"=w666) -> ("error out"=w665:errorcluster, "Device out"=w667:refnum<class "Trigger.lvclass">)  [unwired: 7 in]
          n263 = call-dynamic "Write Trigger.lvclass.vi"("error in (no error)"=w665, "Trigger.lvclass"=w667, "Sync Box in"=w676) -> ("error out"=w673:errorcluster, "Sync Box out"=w675:refnum<class "Sync Box.lvclass">)  [unwired: 7 in]
          n264 = Increment(x=w655) -> (x+1=w654:u32)
          n265 = Select(t=w654, s=w658, f=w655) -> (s? t:f=w657:u32)
          n266 = call-dynamic "Write Sync Box.lvclass.vi"("error in (no error)"=w673, "Sync Box.lvclass"=w675, "SPARC4_AC in"=w674) -> ("error out"=w670:errorcluster, "SPARC4_AC out"=w664:refnum<class "S4ACS_GUI.lvclass">)  [unwired: 7 in]
          n267 = Bundle By Name(cluster=w664, "Obs_state"=w657) -> (w663:refnum<class "S4ACS_GUI.lvclass">)
        }
        frame 306 {
          # "Dispara o comando para o dispositivo corrente."
          n268 = call-dynamic "Read AcquisitionA.vi"("error in (no error)"=w697, "S4ACS_GUI in"=w698) -> ("error out"=w703:errorcluster, "Acquisition.lvclass"=w704:refnum<class "Acquisition.lvclass">, "S4ACS_GUI out"=w700:refnum<class "S4ACS_GUI.lvclass">)  [unwired: 7 in]
          n269 = call-dynamic "Read Channel.vi"("error in (no error)"=w703, "Acquisition in"=w704) -> ("error out"=w692:errorcluster, "Channel.lvclass"=w691:refnum<class "Channel.lvclass">, "Acquisition out"=w702:refnum<class "Acquisition.lvclass">)  [unwired: 7 in]
          n270 = call-dynamic "Read State Machine.vi"("error in (no error)"=w692, "Device in"=w691) -> ("error out"=w693:errorcluster, "State Machine.lvclass"=w695:refnum<class "State Machine.lvclass">, "Device out"=w689:refnum<class "Channel.lvclass">)  [unwired: 7 in]
          n271 = call "Next State.vi"("error in (no error)"=w693, "New_State"=50, "State Machine in"=w695) -> ("error out"=w680:errorcluster, "State Machine out"=w682:refnum<class "State Machine.lvclass">)  [unwired: 7 in]
          n272 = call-dynamic "Write Timer.vi"("error in (no error)"=w680, "Timer"=u32 2, "State Machine in"=w682) -> ("error out"=w679:errorcluster, "State Machine out"=w681:refnum<class "State Machine.lvclass">)  [unwired: 7 in]
          n273 = call-dynamic "Write State Machine.vi"("error in (no error)"=w679, "State Machine.lvclass"=w681, "Device in"=w689) -> ("error out"=w688:errorcluster, "Device out"=w690:refnum<class "Channel.lvclass">)  [unwired: 7 in]
          n274 = Increment(x=w686) -> (x+1=w685:u32)
          n275 = call-dynamic "Write Channel.vi"("error in (no error)"=w688, "Channel.lvclass"=w690, "Acquisition in"=w702) -> ("error out"=w699:errorcluster, "Acquisition out"=w701:refnum<class "Acquisition.lvclass">)  [unwired: 7 in]
          n276 = call-dynamic "Write AcquisitionA.vi"("error in (no error)"=w699, "Acquisition.lvclass"=w701, "S4ACS_GUI in"=w700) -> ("error out"=w696:errorcluster, "S4ACS_GUI out"=w687:refnum<class "S4ACS_GUI.lvclass">)  [unwired: 7 in]
          n277 = Bundle By Name(cluster=w687, "Obs_state"=w685) -> (w684:refnum<class "S4ACS_GUI.lvclass">)
        }
        frame 307 {
          # "Espera terminar a pausa carregada no Timer"
          n278 = call "Read Instrument.lvclass.vi"("error in (no error)"=w721, "S4ACS_GUI in"=w722) -> ("error out"=w727:errorcluster, "Instrument.lvclass"=w728:refnum<class "Instrument.lvclass">, "S4ACS_GUI out"=w724:refnum<class "S4ACS_GUI.lvclass">)  [unwired: 7 in]
          n279 = call "Read WPROT.vi"("error in (no error)"=w727, "Instrument in"=w728) -> ("error out"=w719:errorcluster, "Opt_Selector.lvclass"=w718:refnum<class "Opt_Selector.lvclass">, "Instrument out"=w726:refnum<class "Instrument.lvclass">)  [unwired: 7 in]
          n280 = call-dynamic "Read State Machine.vi"("error in (no error)"=w719, "Device in"=w718) -> ("error out"=w708:errorcluster, "State Machine.lvclass"=w709:refnum<class "State Machine.lvclass">, "Device out"=w716:refnum<class "Opt_Selector.lvclass">)  [unwired: 7 in]
          n281 = Increment(x=w705) -> (x+1=w710:u32)
          n282 = call "Verify Timer.vi"("error in (no error)"=w708, "State Machine in"=w709) -> ("error out"=w706:errorcluster, "timeout"=w711:bool, "State Machine out"=w707:refnum<class "State Machine.lvclass">)  [unwired: 7 in]
          n283 = call-dynamic "Write State Machine.vi"("error in (no error)"=w706, "State Machine.lvclass"=w707, "Device in"=w716) -> ("error out"=w715:errorcluster, "Device out"=w717:refnum<class "Opt_Selector.lvclass">)  [unwired: 7 in]
          n284 = call "Write WPROT.vi"("error in (no error)"=w715, "Opt_Selector.lvclass"=w717, "Instrument in"=w726) -> ("error out"=w723:errorcluster, "Instrument out"=w725:refnum<class "Instrument.lvclass">)  [unwired: 7 in]
          n285 = call "Write Instrument.lvclass.vi"("error in (no error)"=w723, "Instrument.lvclass"=w725, "S4ACS_GUI in"=w724) -> ("error out"=w720:errorcluster, "S4ACS_GUI out"=w714:refnum<class "S4ACS_GUI.lvclass">)  [unwired: 7 in]
          n286 = Select(t=w710, s=w711, f=w705) -> (s? t:f=w712:u32)
          n287 = Bundle By Name(cluster=w714, "Obs_state"=w712) -> (w713:refnum<class "S4ACS_GUI.lvclass">)
        }
        frame 308 {
          # "envia comando TRIGGER para o SyncBox"
          # "Dispara o comando para o dispositivo corrente."
          n288 = call-dynamic "Read Sync Box.lvclass.vi"("error in (no error)"=w745, "SPARC4_AC in"=w746) -> ("error out"=w751:errorcluster, "Sync Box.lvclass"=w731:refnum<class "Sync Box.lvclass">, "SPARC4_AC out"=w748:refnum<class "S4ACS_GUI.lvclass">)  [unwired: 7 in]
          n289 = call-dynamic "Read Trigger.lvclass.vi"("error in (no error)"=w751, "Sync Box in"=w731) -> ("error out"=w740:errorcluster, "Trigger.lvclass"=w739:refnum<class "Trigger.lvclass">, "Sync Box out"=w750:refnum<class "Sync Box.lvclass">)  [unwired: 7 in]
          n290 = call-dynamic "Read State Machine.vi"("error in (no error)"=w740, "Device in"=w739) -> ("error out"=w741:errorcluster, "State Machine.lvclass"=w743:refnum<class "State Machine.lvclass">, "Device out"=w737:refnum<class "Trigger.lvclass">)  [unwired: 7 in]
          n291 = call "Next State.vi"("error in (no error)"=w741, "New_State"=30, "State Machine in"=w743) -> ("error out"=w729:errorcluster, "State Machine out"=w730:refnum<class "State Machine.lvclass">)  [unwired: 7 in]
          n292 = call-dynamic "Write State Machine.vi"("error in (no error)"=w729, "State Machine.lvclass"=w730, "Device in"=w737) -> ("error out"=w736:errorcluster, "Device out"=w738:refnum<class "Trigger.lvclass">)  [unwired: 7 in]
          n293 = Increment(x=w734) -> (x+1=w733:u32)
          n294 = call-dynamic "Write Trigger.lvclass.vi"("error in (no error)"=w736, "Trigger.lvclass"=w738, "Sync Box in"=w750) -> ("error out"=w747:errorcluster, "Sync Box out"=w749:refnum<class "Sync Box.lvclass">)  [unwired: 7 in]
          n295 = call-dynamic "Write Sync Box.lvclass.vi"("error in (no error)"=w747, "Sync Box.lvclass"=w749, "SPARC4_AC in"=w748) -> ("error out"=w744:errorcluster, "SPARC4_AC out"=w735:refnum<class "S4ACS_GUI.lvclass">)  [unwired: 7 in]
          n296 = Bundle By Name(cluster=w735, "Obs_state"=w733) -> (w732:refnum<class "S4ACS_GUI.lvclass">)
        }
        frame 309 {
          # "Espera terminar a execução do comando atual \nantes de ir ao proximo passo da Observação."
          n297 = call-dynamic "Read Sync Box.lvclass.vi"("error in (no error)"=w769, "SPARC4_AC in"=w770) -> ("error out"=w775:errorcluster, "Sync Box.lvclass"=w776:refnum<class "Sync Box.lvclass">, "SPARC4_AC out"=w772:refnum<class "S4ACS_GUI.lvclass">)  [unwired: 7 in]
          n298 = call-dynamic "Read Trigger.lvclass.vi"("error in (no error)"=w775, "Sync Box in"=w776) -> ("error out"=w767:errorcluster, "Trigger.lvclass"=w766:refnum<class "Trigger.lvclass">, "Sync Box out"=w774:refnum<class "Sync Box.lvclass">)  [unwired: 7 in]
          n299 = call-dynamic "Read State Machine.vi"("error in (no error)"=w767, "Device in"=w766) -> ("error out"=w758:errorcluster, "State Machine.lvclass"=w760:refnum<class "State Machine.lvclass">, "Device out"=w764:refnum<class "Trigger.lvclass">)  [unwired: 7 in]
          n300 = call-dynamic "Read State.vi"("error in (no error)"=w758, "State Machine in"=w760) -> ("error out"=w757:errorcluster, "State"=w754:i32, "State Machine out"=w759:refnum<class "State Machine.lvclass">)  [unwired: 7 in]
          n301 = Equal To 0?(x=w754) -> (x = 0?=w756:bool)
          n302 = call-dynamic "Write State Machine.vi"("error in (no error)"=w757, "State Machine.lvclass"=w759, "Device in"=w764) -> ("error out"=w763:errorcluster, "Device out"=w765:refnum<class "Trigger.lvclass">)  [unwired: 7 in]
          n303 = call-dynamic "Write Trigger.lvclass.vi"("error in (no error)"=w763, "Trigger.lvclass"=w765, "Sync Box in"=w774) -> ("error out"=w771:errorcluster, "Sync Box out"=w773:refnum<class "Sync Box.lvclass">)  [unwired: 7 in]
          n304 = Increment(x=w753) -> (x+1=w752:u32)
          n305 = Select(t=w752, s=w756, f=w753) -> (s? t:f=w755:u32)
          n306 = call-dynamic "Write Sync Box.lvclass.vi"("error in (no error)"=w771, "Sync Box.lvclass"=w773, "SPARC4_AC in"=w772) -> ("error out"=w768:errorcluster, "SPARC4_AC out"=w762:refnum<class "S4ACS_GUI.lvclass">)  [unwired: 7 in]
          n307 = Bundle By Name(cluster=w762, "Obs_state"=w755) -> (w761:refnum<class "S4ACS_GUI.lvclass">)
        }
        frame 310 {
          # "Espera terminar a execução do comando atual \nantes de ir ao proximo passo da Observação."
          n308 = call-dynamic "Read AcquisitionA.vi"("error in (no error)"=w794, "S4ACS_GUI in"=w795) -> ("error out"=w800:errorcluster, "Acquisition.lvclass"=w801:refnum<class "Acquisition.lvclass">, "S4ACS_GUI out"=w797:refnum<class "S4ACS_GUI.lvclass">)  [unwired: 7 in]
          n309 = call-dynamic "Read Channel.vi"("error in (no error)"=w800, "Acquisition in"=w801) -> ("error out"=w792:errorcluster, "Channel.lvclass"=w791:refnum<class "Channel.lvclass">, "Acquisition out"=w799:refnum<class "Acquisition.lvclass">)  [unwired: 7 in]
          n310 = call-dynamic "Read State Machine.vi"("error in (no error)"=w792, "Device in"=w791) -> ("error out"=w783:errorcluster, "State Machine.lvclass"=w785:refnum<class "State Machine.lvclass">, "Device out"=w789:refnum<class "Channel.lvclass">)  [unwired: 7 in]
          n311 = call-dynamic "Read State.vi"("error in (no error)"=w783, "State Machine in"=w785) -> ("error out"=w782:errorcluster, "State"=w779:i32, "State Machine out"=w784:refnum<class "State Machine.lvclass">)  [unwired: 7 in]
          n312 = Equal To 0?(x=w779) -> (x = 0?=w781:bool)
          n313 = call-dynamic "Write State Machine.vi"("error in (no error)"=w782, "State Machine.lvclass"=w784, "Device in"=w789) -> ("error out"=w788:errorcluster, "Device out"=w790:refnum<class "Channel.lvclass">)  [unwired: 7 in]
          n314 = call-dynamic "Write Channel.vi"("error in (no error)"=w788, "Channel.lvclass"=w790, "Acquisition in"=w799) -> ("error out"=w796:errorcluster, "Acquisition out"=w798:refnum<class "Acquisition.lvclass">)  [unwired: 7 in]
          n315 = Select(t=u32 301, s=w781, f=w778) -> (s? t:f=w780:u32)
          n316 = call-dynamic "Write AcquisitionA.vi"("error in (no error)"=w796, "Acquisition.lvclass"=w798, "S4ACS_GUI in"=w797) -> ("error out"=w793:errorcluster, "S4ACS_GUI out"=w787:refnum<class "S4ACS_GUI.lvclass">)  [unwired: 7 in]
          n317 = Bundle By Name(cluster=w787, "Obs_state"=w780) -> (w786:refnum<class "S4ACS_GUI.lvclass">)
        }
        frame 311 {
          n318 = call-dynamic "Read ciclos.vi"("error in (no error)"=w814, "S4ACS_GUI in"=w815) -> ("error out"=w803:errorcluster, "ciclos"=w808:u32, "S4ACS_GUI out"=w816:refnum<class "S4ACS_GUI.lvclass">)  [unwired: 7 in]
          n319 = Decrement(x=w808) -> (x-1=w802:u32)
          n320 = Greater Than 0?(x=w802) -> (x > 0?=w809:bool)
          n321 = case shown="False" w809 {
            selector: w809 -> [w818 w820]
            tunnel: w802 -> [_ w819]
            tunnel: [w818 w820] -> w807
            tunnel: [u32 0 w819] -> w804
            frame False {
            }
            frame True {
            }
          }
          n322 = Select(t=u32 301, s=w807, f=u32 0) -> (s? t:f=w810:u32)
          n323 = call-dynamic "Write ciclos.vi"("error in (no error)"=w803, "ciclos"=w804, "S4ACS_GUI in"=w816) -> ("error out"=w813:errorcluster, "S4ACS_GUI out"=w812:refnum<class "S4ACS_GUI.lvclass">)  [unwired: 7 in]
          n324 = Bundle By Name(cluster=w812, "Obs_state"=w810) -> (w811:refnum<class "S4ACS_GUI.lvclass">)
        }
        frame 400 {
          # "Estado de \"PAUSE\": não faz nada aqui até que o botão Start SM seja pressionado para continuar o loop de HandleObservation.vi"
        }
      }
    }
    frame Error {
    }
  }
  "error out" <- w3
  "S4ACS_GUI out" <- w1
